vi "Flow Modelling_Comparison_Virtual Subjects_V2.4.1.vi"() -> ()   [LabVIEW 2017]
uses:
  <vilib>/Utility/file.llb/Read Delimited Spreadsheet (DBL).vi
  <vilib>/Analysis/NI_AALPro.lvlib
  <vilib>/gmath/NI_Gmath.lvlib
  <vilib>/Analysis/NI_AALBase.lvlib
  <vilib>/Analysis/baseanly.llb/Mean (DBL).vi
  <vilib>/Analysis/NI_AAL_SigProc.lvlib
panel:
  out "Array":dbl[][](array[numeric])
  out "mean 2":dbl
  out "SDW ZC 2":dbl
  out "mean":dbl
  in  "Min seperation B/W peaks":dbl format="%#_13g"
  out "intercept":dbl
  out "slope":dbl
  out "A1/A2":dbl
  out "Age (years)":dbl=75.0
  out "True - Type A or B":bool
  in  "Save Data":bool
  out "Saving Data":bool
  out "Loop time (ms)":u32=22
  in  "Loop Condition":bool
  in  "Loop Wait Time (ms)":u32
  in  "Start Subject ID":i32=1
  in  "Last Sub ID":i32=1000
  out "Current ID":i32=4341
  in  "Tab Control":T1(tab)
  out "Flow Rate":waveform(dbl)(graph)={"t0"=timestamp(0 s since 1904-01-01), "dt"=0.002, "Y"=array[402 elements]}
  in  "FileName P":string(combo)="PWs_Carotid_P.csv"
  in  "Param Folder Path":path=path "F:/HTIC Works/Cardiovascular Research/Data Set/Virtual Subjects Database"
  in  "Folder  Path":path=path "F:/HTIC Works/Cardiovascular Research/Data Set/Virtual Subjects Database/Virtual Subjects Database CSV"
  out "Hemodynamic Param":dbl[](array[numeric])=[75.0, 74.442, 66.405, 4.9433, 302.0, 1083.3, 80.0, 0.71264, 142.52, 52.007, 95.245, 90.517, 145.8, 50.057, 94.967, 95.743, 1.0577, 44.782, 49.473, 62.0, 12.106, 12.84, 15.216, 14.693, 38.642, 25.707, 15.209, 9.2134, 112.02, 2.665, 7.9438, 154.14]
  in  "Original Sampling Rate (Hz)":dbl=500.0
  in  "Re Sample?":bool
  out "dt":dbl=0.002
  in  "Re Sample Rate(Hz)":dbl=500.0 format="%#_13g"
  out "Pressure":waveform(dbl)(graph)={"t0"=timestamp(0 s since 1904-01-01), "dt"=0.002, "Y"=array[402 elements]}
  in  "FileName U":string(combo)="PWs_Carotid_U.csv"
  in  "FileName A":string(combo)="PWs_Carotid_A.csv"
  in  "FileName PPG":string(combo)="PWs_Carotid_PPG.csv"
  out "Flow Velocity":waveform(dbl)(graph)={"t0"=timestamp(0 s since 1904-01-01), "dt"=0.002, "Y"=array[402 elements]}
  out "Diameter":waveform(dbl)(graph)={"t0"=timestamp(0 s since 1904-01-01), "dt"=0.002, "Y"=array[402 elements]}
  out "PPG":waveform(dbl)(graph)={"t0"=timestamp(0 s since 1904-01-01), "dt"=0.002, "Y"=array[402 elements]}
  in  "FileName Param":string(combo)="pwdb_haemod_params.csv"
  out "Area":waveform(dbl)(graph)={"t0"=timestamp(0 s since 1904-01-01), "dt"=0.002, "Y"=array[402 elements]}
  in  "File to Save Data":path=path "F:/HTIC Works/Cardiovascular Research/Analysis and Results/Flow Model Comparison Virtual Subjects/Journal Data Analysis V2.0/Carotid_Flow_2_Ray_Type_Based_Master_0001_1000.xlsx" caption="Filename"
  out "Derivatives of P(t) 2":dynamicdata(graph)=[{"t0"=timestamp(0 s since 1904-01-01), "dt"=0.002, "Y"=array[402 elements]}, {"t0"=timestamp(0 s since 1904-01-01), "dt"=0.002, "Y"=array[402 elements]}, {"t0"=timestamp(0 s since 1904-01-01), "dt"=0.002, "Y"=array[402 elements]}, {"t0"=timestamp(0 s since 1904-01-01), "dt"=0.002, "Y"=array[402 elements]}, {"t0"=timestamp(0 s since 1904-01-01), "dt"=0.002, "Y"=array[402 elements]}, {"t0"=timestamp(0 s since 1904-01-01), "dt"=0.002, "Y"=[nan, nan, nan, nan, nan, 58.29028179551122, nan, nan, nan, nan, nan, nan, nan, nan, nan, nan, nan, 82.59575810473817, nan, nan, 88.92912718204488, 91.05758354114712, nan, nan, nan, nan, nan, nan, nan, nan, nan, nan, nan, nan, nan, nan, nan, nan, nan, nan, nan, 118.08771072319202, nan, nan, nan, 121.945536159601, nan, nan, nan, nan, nan, nan, nan, nan, nan, nan, nan, nan, nan, nan, nan, nan, nan, nan, nan, nan, nan, nan, nan, nan, nan, nan, nan, nan, nan, nan, nan, nan, nan, nan, nan, nan, nan, nan, nan, nan, nan, nan, nan, nan, nan, nan, nan, 143.88944139650874, 143.89889775561096, nan, nan, nan, nan, nan, nan, nan, nan, nan, nan, nan, nan, nan, nan, nan, nan, nan, nan, nan, nan, nan, nan, nan, nan, nan, nan, nan, nan, nan, nan, nan, nan, nan, nan, nan, nan, nan, nan, nan, nan, nan, nan, nan, nan, nan, nan, nan, nan, nan, nan, nan, nan, nan, nan, nan, nan, nan, nan, nan, nan, nan, nan, nan, nan, nan, 114.8030174563591, nan, nan, nan, nan, nan, nan, nan, nan, nan, nan, nan, nan, nan, nan, nan, nan, nan, nan, nan, nan, nan, nan, nan, nan, nan, nan, nan, nan, nan, nan, nan, nan, nan, nan, nan, nan, nan, nan, nan, nan, nan, nan, nan, nan, nan, nan, nan, nan, nan, nan, nan, nan, nan, nan, nan, nan, nan, nan, nan, nan, nan, nan, nan, nan, nan, nan, nan, nan, nan, nan, nan, nan, nan, nan, nan, nan, nan, nan, nan, nan, nan, nan, nan, nan, nan, nan, nan, nan, nan, nan, nan, nan, nan, nan, nan, nan, nan, nan, nan, nan, nan, nan, nan, nan, nan, nan, nan, nan, nan, nan, nan, nan, nan, nan, nan, nan, nan, nan, nan, nan, nan, nan, nan, nan, nan, nan, nan, nan, nan, nan, nan, nan, nan, nan, nan, nan, nan, nan, nan, nan, nan, nan, nan, nan, nan, nan, nan, nan, nan, nan, nan, nan, nan, nan, nan, nan, nan, nan, nan, nan, nan, nan, nan, nan, nan, nan, nan, nan, nan, nan, nan, nan, nan, nan, nan, nan, nan, nan, nan, nan, nan, nan, nan, nan, nan, nan, nan, nan, nan, nan, nan, nan, nan, nan, nan, nan, nan, nan, nan, nan, nan, nan, nan, nan, nan, nan, nan, nan, nan, nan, nan, nan, nan, nan, nan, nan, nan, nan, nan, nan, nan, nan, nan, nan, nan, nan, nan, nan, nan, nan, nan, nan, nan, nan, nan, nan, nan, nan, nan, nan, nan]}]
  in  "Derivative LPF cutoff (Hz)":dbl=75.0
  in  "SG Filter Config":T2={"polynomial order"=4, "side points"=28.0}
  out "Derivatives of P(t)":dynamicdata(graph)=[{"t0"=timestamp(0 s since 1904-01-01), "dt"=0.002, "Y"=array[402 elements]}, {"t0"=timestamp(0 s since 1904-01-01), "dt"=0.002, "Y"=array[401 elements]}, {"t0"=timestamp(0 s since 1904-01-01), "dt"=0.002, "Y"=array[401 elements]}, {"t0"=timestamp(0 s since 1904-01-01), "dt"=0.002, "Y"=array[401 elements]}, {"t0"=timestamp(0 s since 1904-01-01), "dt"=0.002, "Y"=array[402 elements]}, {"t0"=timestamp(0 s since 1904-01-01), "dt"=0.002, "Y"=[nan, nan, nan, nan, nan, 58.29028179551122, nan, nan, nan, nan, nan, nan, nan, nan, nan, nan, nan, 82.59575810473817, nan, nan, 88.92912718204488, 91.05758354114712, nan, nan, nan, nan, nan, nan, nan, nan, nan, nan, nan, nan, nan, nan, nan, nan, nan, nan, nan, 118.08771072319202, nan, nan, nan, 121.945536159601, nan, nan, nan, nan, nan, nan, nan, nan, nan, nan, nan, nan, nan, nan, nan, nan, nan, nan, nan, nan, nan, nan, nan, nan, nan, nan, nan, nan, nan, nan, nan, nan, nan, nan, nan, nan, nan, nan, nan, nan, nan, nan, nan, nan, nan, nan, nan, 143.88944139650874, 143.89889775561096, nan, nan, nan, nan, nan, nan, nan, nan, nan, nan, nan, nan, nan, nan, nan, nan, nan, nan, nan, nan, nan, nan, nan, nan, nan, nan, nan, nan, nan, nan, nan, nan, nan, nan, nan, nan, nan, nan, nan, nan, nan, nan, nan, nan, nan, nan, nan, nan, nan, nan, nan, nan, nan, nan, nan, nan, nan, nan, nan, nan, nan, nan, nan, nan, nan, 114.8030174563591, nan, nan, nan, nan, nan, nan, nan, nan, nan, nan, nan, nan, nan, nan, nan, nan, nan, nan, nan, nan, nan, nan, nan, nan, nan, nan, nan, nan, nan, nan, nan, nan, nan, nan, nan, nan, nan, nan, nan, nan, nan, nan, nan, nan, nan, nan, nan, nan, nan, nan, nan, nan, nan, nan, nan, nan, nan, nan, nan, nan, nan, nan, nan, nan, nan, nan, nan, nan, nan, nan, nan, nan, nan, nan, nan, nan, nan, nan, nan, nan, nan, nan, nan, nan, nan, nan, nan, nan, nan, nan, nan, nan, nan, nan, nan, nan, nan, nan, nan, nan, nan, nan, nan, nan, nan, nan, nan, nan, nan, nan, nan, nan, nan, nan, nan, nan, nan, nan, nan, nan, nan, nan, nan, nan, nan, nan, nan, nan, nan, nan, nan, nan, nan, nan, nan, nan, nan, nan, nan, nan, nan, nan, nan, nan, nan, nan, nan, nan, nan, nan, nan, nan, nan, nan, nan, nan, nan, nan, nan, nan, nan, nan, nan, nan, nan, nan, nan, nan, nan, nan, nan, nan, nan, nan, nan, nan, nan, nan, nan, nan, nan, nan, nan, nan, nan, nan, nan, nan, nan, nan, nan, nan, nan, nan, nan, nan, nan, nan, nan, nan, nan, nan, nan, nan, nan, nan, nan, nan, nan, nan, nan, nan, nan, nan, nan, nan, nan, nan, nan, nan, nan, nan, nan, nan, nan, nan, nan, nan, nan, nan, nan, nan, nan, nan, nan, nan, nan, nan, nan, nan, nan]}]
  out "Fid. Points":T3={"MX (sec)"=0.188, "FDW/SDW ZC (sec)"=0.058, "FoDW ZC (sec)"=0.12, "IP (sec)"=0.23573963204691295, "DN (sec)"=0.3188943360526481}
  out "True Flow Peak (sec)":dbl=0.042
  out "Peak of FoDW":dbl[](array[numeric])
  out "Fid. Points (SDW)":T4
  out "Zc (mmHg/ml/s)":dbl=1.725966148386607
  out "PVR (mmHg/ml/s)":dbl=16.50058753410355
  out "Input Impedence - Phase Spectrum":waveform(dbl)(graph)={"t0"=timestamp(0 s since 1904-01-01), "dt"=1.243781094527363, "Y"=array[402 elements]}
  out "Input Impedence - Magnitude Spectrum":waveform(dbl)(graph)={"t0"=timestamp(0 s since 1904-01-01), "dt"=1.243781094527363, "Y"=array[402 elements]}
  in  "Settings":T5={"Min. Harmonics for Zc"=4.0, "Max. Harmonics for Zc"=10.0}
  out "PWV (dPdU) (m/s)":dbl=21.61401999257581
  out "PWV (BH) (m/s)":dbl=13.16463528929057
  out "Zc (mmHg/ml/s)":dbl=2.673030331101323
  out "Zc (mmHg/ml/s)":dbl=1.6280853556278632
  in  "Settings 2":T6={"Min. Hrmonic for Zc"=4.0, "Max. Harmonic for Zc"=10.0}
  out "Input Impedence - Magnitude Spectrum  2":waveform(dbl)(graph)={"t0"=timestamp(0 s since 1904-01-01), "dt"=1.243781094527363, "Y"=array[402 elements]}
  out "WSA Q - Time Domain":dynamicdata(graph)=[{"t0"=timestamp(0 s since 1904-01-01), "dt"=0.002, "Y"=array[402 elements]}, {"t0"=timestamp(0 s since 1904-01-01), "dt"=0.002, "Y"=array[402 elements]}, {"t0"=timestamp(0 s since 1904-01-01), "dt"=0.002, "Y"=array[402 elements]}]
  out "WSA P - Time. Domain":dynamicdata(graph)=[{"t0"=timestamp(0 s since 1904-01-01), "dt"=0.002, "Y"=array[402 elements]}, {"t0"=timestamp(0 s since 1904-01-01), "dt"=0.002, "Y"=array[402 elements]}, {"t0"=timestamp(0 s since 1904-01-01), "dt"=0.002, "Y"=array[402 elements]}]
  out "WSA Q - Freq. Domain":dynamicdata(graph)=[{"t0"=timestamp(0 s since 1904-01-01), "dt"=0.002, "Y"=array[402 elements]}, {"t0"=timestamp(0 s since 1904-01-01), "dt"=0.002, "Y"=array[402 elements]}, {"t0"=timestamp(0 s since 1904-01-01), "dt"=0.002, "Y"=array[402 elements]}]
  out "WSA P - Freq. Domain":dynamicdata(graph)=[{"t0"=timestamp(0 s since 1904-01-01), "dt"=0.002, "Y"=array[402 elements]}, {"t0"=timestamp(0 s since 1904-01-01), "dt"=0.002, "Y"=array[402 elements]}, {"t0"=timestamp(0 s since 1904-01-01), "dt"=0.002, "Y"=array[402 elements]}]
  out "Reflection Markers\n(Time Domain WSA)":T7={"del Pf"=58.89527020287039, "del Pb"=41.94891474189147, "RM"=0.7122628794705317, "RI (%)"=41.59775277560059}
  out "Reflection Markers\n(Freq. Domain WSA)":T7={"del Pf"=54.396213288918176, "del Pb"=39.3327759196838, "RM"=0.7230793016928043, "RI (%)"=41.96436582938637}
  out "m-Ray":dbl[][](graph)
  out "Magnitude Spectrum Flow":dynamicdata(graph)=[{"t0"=timestamp(0 s since 1904-01-01), "dt"=1.243781094527363, "Y"=array[201 elements]}, {"t0"=timestamp(0 s since 1904-01-01), "dt"=1.2468827930174562, "Y"=[2.875475307707561, 3.6127603544098683, 2.601261591287198, 1.6917776838030885, 1.1941771538443262, 0.9487554465134683, 0.7694402798879594, 0.6103288199328872, 0.4731880654990021, 0.36211255149969857, 0.2769548748250606, 0.21434413683079837, 0.1694301710225544, 0.13733282803274616, 0.11402801928183168, 0.09662400462795698, 0.08321657451570393, 0.07259766150124436, 0.0639964187444626, 0.056904741290042034, 0.050973683000770764, 0.04595437718864926, 0.041663805403745764, 0.037964077971374716, 0.03474926453416704, 0.031936660619215164, 0.029460797434445064, 0.027269222135548016, 0.025319459881613045, 0.023576786205464897, 0.022012567439413037, 0.020603006949110554, 0.019328186072354925, 0.018171322213655604, 0.017118189050174, 0.016156659190830255, 0.015276340329362368, 0.014468283485487652, 0.013724747334456168, 0.013039006543154078, 0.012405194902865806, 0.011818176176362818, 0.011273437168463712, 0.010766998730631047, 0.010295341324676783, 0.009855342472415885, 0.009444223960556648, 0.009059507092347416, 0.008698974608396304, 0.008360638159887837, 0.008042710424359204, 0.007743581119138634, 0.0074617962998756145, 0.007196040438151105, 0.006945120858491341, 0.006707954185289361, 0.006483554507505954, 0.00627102301606209, 0.006069538907604141, 0.005878351380350117, 0.005696772574338759, 0.005524171330542793, 0.005359967661818076, 0.0052036278441806956, 0.00505466004996289, 0.0049126104554011564, 0.0047770597645341445, 0.004647620099193955, 0.004523932211592496, 0.004405662981762424, 0.004292503166987805, 0.004184165374607464, 0.004080382233152479, 0.00398090473991798, 0.0038855007657562566, 0.0037939537001872204, 0.003706061221966357, 0.0036216341819848476, 0.003540495586902267, 0.0034624796732586217, 0.003387431062954797, 0.0033152039920320057, 0.003245661605543917, 0.003178675312137021, 0.0031141241926116317, 0.0030518944573612915, 0.002991878948129061, 0.0029339766799803533, 0.002878092419823849, 0.0028241362981836623, 0.0027720234512541744, 0.002721673690565746, 0.002673011197849946, 0.002625964242935183, 0.0025804649226975913, 0.0025364489192982675, 0.0024938552760841457, 0.002452626189704618, 0.0024127068171034462, 0.002374045096189568, 0.0023365915790872476, 0.00230029927696597, 0.0022651235155401643, 0.00223102180040995, 0.002197953691483903, 0.0021658806857857635, 0.0021347661080214518, 0.0021045750083141137, 0.002075274066582661, 0.002046831503073918, 0.002019216994597034, 0.001992401596055293, 0.0019663576668881018, 0.0019410588020834878, 0.0019164797674358094, 0.0018925964387492304, 0.0018693857447258516, 0.0018468256132752187, 0.001824894921018906, 0.0018035734457731835, 0.0017828418218158767, 0.001762681497743173, 0.0017430746967612542, 0.0017240043792384348, 0.0017054542073845459, 0.0016874085119173083, 0.0016698522605864423, 0.001652771028445564, 0.0016361509697526123, 0.0016199787914136649, 0.0016042417278542903, 0.001588927517255393, 0.0015740243790484032, 0.0015595209926116604, 0.0015454064770874616, 0.00153167037225232, 0.001518302620390819, 0.0015052935490970777, 0.0014926338549648165, 0.0014803145881091097, 0.0014683271374716065, 0.0014566632168709034, 0.0014453148517466628, 0.0014342743665710113, 0.001423534372880088, 0.0014130877578963801, 0.0014029276737148768, 0.0013930475270104972, 0.0013834409692506475, 0.0013741018873806075, 0.0013650243949579809, 0.0013562028237132488, 0.001347631715514795, 0.001339305814715998, 0.001331220060867736, 0.0013233695817755878, 0.0013157496868858958, 0.0013083558609843034, 0.0013011837581918626, 0.0012942291962411733, 0.001287488151027233, 0.0012809567514092683, 0.0012746312742586898, 0.001268508139743941, 0.0012625839068313555, 0.0012568552690039238, 0.0012513190501797634, 0.0012459722008272467, 0.0012408117942623747, 0.0012358350231262449, 0.0012310391960329112, 0.0012264217343779297, 0.0012219801693055961, 0.0012177121388237048, 0.0012136153850642354, 0.0012096877516847855, 0.0012059271813955653, 0.0012023317136246772, 0.0011988994822993734, 0.001195628713749398, 0.0011925177247257275, 0.0011895649205306458, 0.0011867687932546778, 0.0011841279201161216, 0.0011816409619078844, 0.0011793066615325718, 0.0011771238426436684, 0.0011750914083724123, 0.0011732083401441626, 0.0011714736965906787, 0.0011698866125403051, 0.0011684462980971273, 0.0011671520378015504, 0.001166003189871259, 0.0011649991855236896, 0.0011641395283739614, 0.0011634237939147955, 0.001162851629066894, 0.0011624227518108622, 0.0011621369508905742]}, {"t0"=timestamp(0 s since 1904-01-01), "dt"=1.2468827930174562, "Y"=[3.7508500728179532, 4.5245622515687804, 2.7381315525642167, 1.2960200155292345, 1.0722958286591062, 0.8591503498715637, 0.5835761351400733, 0.5409096008292368, 0.4147688861808805, 0.32048488221512145, 0.29183680892133157, 0.20830482531413225, 0.17423818235279553, 0.14408511660630235, 0.09295183114010737, 0.08066585123213792, 0.05245806743771004, 0.02590171014916199, 0.020442136353742146, 0.009784595168948028, 0.011474868149847212, 0.018825340120545746, 0.03141941850998123, 0.02947371209902249, 0.03581015185540728, 0.03916182600261739, 0.034561584685847385, 0.03873980795285254, 0.03511313154107394, 0.03116123233701509, 0.031912924558875844, 0.02491230464070535, 0.022634935322990154, 0.020002838241100496, 0.012977935928489096, 0.011842854009855807, 0.007328558363566402, 0.002244810549003913, 0.0017397365874485381, 0.004532861640760953, 0.005726147321061923, 0.007405227865666979, 0.010966826405368063, 0.010414787796708059, 0.012306490583137283, 0.013401593295404544, 0.011949767607856616, 0.013387475714232414, 0.012171390141769123, 0.01081417184514539, 0.011125760149963679, 0.008526081768583077, 0.007706560831230049, 0.006699089826276321, 0.0039008866101970107, 0.003497414628569744, 0.001773368465099045, 0.00047989313530877586, 0.000946729075561772, 0.003251762903982372, 0.0038078559422530457, 0.004464019719007958, 0.006079369674982631, 0.005710634319960984, 0.006535479575465597, 0.006978137171141666, 0.006151608672064754, 0.006802070499646614, 0.006078711193183457, 0.00530783478093735, 0.005407263205985483, 0.003953597615943812, 0.0034948522720437136, 0.002903582890828807, 0.0013417822627342514, 0.0011393625525869247, 0.0005372069831318354, 0.0010815373739305463, 0.0012525598901868763, 0.002571610507446599, 0.002850884833977321, 0.003162498326287775, 0.004062517723188385, 0.0037524296049899404, 0.0041825485685056596, 0.004367767696673512, 0.0037782933874932045, 0.0041208391029226256, 0.0035852324475160046, 0.003052998354699827, 0.003063478402111416, 0.0020799201132795865, 0.0017818005793410658, 0.001359917731252523, 0.00033081700568838695, 0.0002472925184793049, 0.0006353239473414299, 0.001224390605035756, 0.001291746507604338, 0.002145466179865607, 0.002283235237248078, 0.0024430485314186428, 0.003006307934302749, 0.0027230010421153443, 0.0029731708270343696, 0.0030340432764327826, 0.002564428140558709, 0.002763719020567095, 0.0023209272461199855, 0.001917753419707948, 0.0018866915958778356, 0.001142184536290282, 0.0009435979213443637, 0.0006009834971304799, 0.00015563871856385234, 0.00025488504953471, 0.0007999141673041498, 0.0012400965762612182, 0.0012548964511063009, 0.0018618021285207076, 0.00191633817055137, 0.0019995049706351274, 0.002379614848642651, 0.0021097458485435615, 0.0022683889315689384, 0.0022593891694644755, 0.0018602703564758424, 0.001985640883157327, 0.0015932606855256976, 0.0012728288480013971, 0.0012185033302108954, 0.000609944887714449, 0.0004946215828014669, 0.00017913489638318402, 0.00041534120526386884, 0.00046290996057953346, 0.0008937400922277749, 0.0012240257805451386, 0.0012081530224320456, 0.0016724486765397817, 0.0016718389500814865, 0.0017138288795263978, 0.001984171073359226, 0.0017196672622895987, 0.001829264129194719, 0.001774799824540436, 0.0014202635123030359, 0.0015044633021834733, 0.0011381144596961585, 0.000877372347329584, 0.0008050885390449594, 0.000278499702809272, 0.0002698473312872596, 9.641728518399287e-05, 0.0005793341438433319, 0.0005960928699227096, 0.0009585113628025477, 0.0012121650203852962, 0.001177123910926902, 0.0015550836888611236, 0.0015134003492032705, 0.0015330199512812203, 0.001732245289408295, 0.0014663755863387655, 0.0015491377483849418, 0.0014597230614821599, 0.001133181926904543, 0.0011921630821759533, 0.0008345755925252025, 0.0006210987382223606, 0.0005288786284448412, 6.866564153260373e-05, 0.0002348812509856483, 0.0002819154758607105, 0.0007052224535725401, 0.0006992791072680399, 0.0010249158270583772, 0.0012232930978217363, 0.0011755815989433625, 0.0015004968361050067, 0.001423993327248736, 0.001431481248622589, 0.0015808000227044321, 0.0013062342066300684, 0.0013737589587263772, 0.0012521900650118711, 0.0009403417096469833, 0.0009811026261219574, 0.0006175136507945863, 0.00044542496927388764, 0.00032548202569685256, 0.00015424392272724206, 0.00031738262133868103, 0.00044468091725355797, 0.0008292865567833156, 0.0008050655206424677, 0.0011156902134628515, 0.0012719611413126496, 0.0012146041020032518, 0.0015074412858806026]}]
  out "RMSE Ray Model":dbl=4.137711413874004
  out "Model Error (ms)":dbl[](array[numeric])=[5.999999999999998, 4.029709151279315]
  out "Reference Flow Rate":T8={"Flow Peak (sec)"=0.042, "Flow Peak (Amp)"=18.5690232}
  out "Flow Rate Model":dynamicdata(graph)=[{"t0"=timestamp(0 s since 1904-01-01), "dt"=0.002, "Y"=array[402 elements]}, {"t0"=timestamp(0 s since 1904-01-01), "dt"=0.002, "Y"=[nan, nan, nan, nan, nan, nan, nan, nan, nan, nan, nan, nan, nan, nan, nan, nan, nan, nan, nan, nan, 88.92912718204488, nan, nan, nan, nan, nan, nan, nan, nan, nan, nan, nan, nan, nan, nan, nan, nan, nan, nan, nan, nan, nan, nan, nan, nan, nan, nan, nan, nan, nan, nan, nan, nan, nan, nan, nan, nan, nan, nan, nan, nan, nan, nan, nan, nan, nan, nan, nan, nan, nan, nan, nan, nan, nan, nan, nan, nan, nan, nan, nan, nan, nan, nan, nan, nan, nan, nan, nan, nan, nan, nan, nan, nan, nan, nan, nan, nan, nan, nan, nan, nan, nan, nan, nan, nan, nan, nan, nan, nan, nan, nan, nan, nan, nan, nan, nan, nan, nan, nan, nan, nan, nan, nan, nan, nan, nan, nan, nan, nan, nan, nan, nan, nan, nan, nan, nan, nan, nan, nan, nan, nan, nan, nan, nan, nan, nan, nan, nan, nan, nan, nan, nan, nan, nan, nan, nan, nan, nan, nan, nan, 114.8030174563591, nan, nan, nan, nan, nan, nan, nan, nan, nan, nan, nan, nan, nan, nan, nan, nan, nan, nan, nan, nan, nan, nan, nan, nan, nan, nan, nan, nan, nan, nan, nan, nan, nan, nan, nan, nan, nan, nan, nan, nan, nan, nan, nan, nan, nan, nan, nan, nan, nan, nan, nan, nan, nan, nan, nan, nan, nan, nan, nan, nan, nan, nan, nan, nan, nan, nan, nan, nan, nan, nan, nan, nan, nan, nan, nan, nan, nan, nan, nan, nan, nan, nan, nan, nan, nan, nan, nan, nan, nan, nan, nan, nan, nan, nan, nan, nan, nan, nan, nan, nan, nan, nan, nan, nan, nan, nan, nan, nan, nan, nan, nan, nan, nan, nan, nan, nan, nan, nan, nan, nan, nan, nan, nan, nan, nan, nan, nan, nan, nan, nan, nan, nan, nan, nan, nan, nan, nan, nan, nan, nan, nan, nan, nan, nan, nan, nan, nan, nan, nan, nan, nan, nan, nan, nan, nan, nan, nan, nan, nan, nan, nan, nan, nan, nan, nan, nan, nan, nan, nan, nan, nan, nan, nan, nan, nan, nan, nan, nan, nan, nan, nan, nan, nan, nan, nan, nan, nan, nan, nan, nan, nan, nan, nan, nan, nan, nan, nan, nan, nan, nan, nan, nan, nan, nan, nan, nan, nan, nan, nan, nan, nan, nan, nan, nan, nan, nan, nan, nan, nan, nan, nan, nan, nan, nan, nan, nan, nan, nan, nan, nan, nan, nan, nan, nan, nan, nan, nan, nan, nan, nan, nan]}, {"t0"=timestamp(0 s since 1904-01-01), "dt"=0.002, "Y"=array[402 elements]}, {"t0"=timestamp(0 s since 1904-01-01), "dt"=0.002, "Y"=array[401 elements]}, {"t0"=timestamp(0 s since 1904-01-01), "dt"=0.002, "Y"=array[401 elements]}, {"t0"=timestamp(0 s since 1904-01-01), "dt"=0.002, "Y"=array[401 elements]}]
  out "T_Ejection Period (sec)":dbl=0.31908927539190324
  out "T_Flow Peak (sec)":dbl=0.04
  out "Model Optimised Parameter":dbl[](array[numeric])=[0.10000000149011612, 0.03999999910593033]
  out "#Rayeligh":dbl=2.0
  out "correlation coefficient r":dbl=0.9951884045954855 format="%.7g"
  out "Amplitude":dbl[](array[numeric])
  out "A2/A1":dbl
  in  "A2/A1 2":dbl
  out "m-Ray RWTT XCorr (TD)(ms)":dbl=72.00000000000001
  out "Ref. RWTT XCorr (TD)(ms)":dbl=48.0
  out "Tri.  RWTT XCorr (TD)(ms)":dbl=84.0
  out "m-Ray RWTT XCorr (FD)(ms)":dbl=42.0
  out "Ref. RWTT XCorr (FD)(ms)":dbl=34.0
  out "Tri.  RWTT XCorr (FD)(ms)":dbl=48.0
  out "m-Ray RWTT ZC (TD)(ms)":dbl=72.41752223636087
  out "Ref. RWTT ZC (TD)(ms)":dbl=48.9881513554138
  out "Tri.  RWTT  ZC (TD)(ms)":dbl=79.1625821471164
  out "m-Ray RWTT ZC (FD)(ms)":dbl=46.35509024365538
  out "Ref. RWTT ZC (FD)(ms)":dbl=36.51530586869714
  out "Tri.  RWTT ZC (FD)(ms)":dbl=48.6059655733487
  out "RMSE (Fwd Triangular TD)":dbl=3.386520035598584
  out "RMSE (Bwd Rayleigh TD)":dbl=3.726988173192518
  out "RMSE (Fwd Rayleigh TD)":dbl=3.726988173192517
  out "RMSE (Bwd Triangular TD)":dbl=3.3865200355985845
  out "Backward Pressure Wave (Time Domain Analysis)":dynamicdata(graph)=[{"t0"=timestamp(0 s since 1904-01-01), "dt"=0.002, "Y"=array[402 elements]}, {"t0"=timestamp(0 s since 1904-01-01), "dt"=0.002, "Y"=array[401 elements]}, {"t0"=timestamp(0 s since 1904-01-01), "dt"=0.002, "Y"=array[401 elements]}]
  out "Forward Pressure Wave (Time Domain Analysis)":dynamicdata(graph)=[{"t0"=timestamp(0 s since 1904-01-01), "dt"=0.002, "Y"=array[402 elements]}, {"t0"=timestamp(0 s since 1904-01-01), "dt"=0.002, "Y"=array[401 elements]}, {"t0"=timestamp(0 s since 1904-01-01), "dt"=0.002, "Y"=array[401 elements]}]
  out "Rayleigh (FD)":T7={"del Pf"=50.48708754008288, "del Pb"=45.11476622884561, "RM"=0.8935901916114282, "RI (%)"=47.19026300252385}
  out "Triangular (FD)":T7={"del Pf"=54.83519661326886, "del Pb"=40.555492402948346, "RM"=0.739588711406842, "RI (%)"=42.51514777931164}
  out "Reference (FD)":T7={"del Pf"=54.396213288918176, "del Pb"=39.3327759196838, "RM"=0.7230793016928043, "RI (%)"=41.96436582938637}
  out "RMSE (Fwd Triangular FD)":dbl=1.7174517386171273
  out "RMSE (Bwd Rayleigh FD)":dbl=2.4763715027755246
  out "RMSE (Fwd Rayleigh FD)":dbl=2.476371502775524
  out "RMSE (Bwd Triangular FD)":dbl=1.7174517386171277
  out "Backward Pressure Wave (Freq. Domain Analysis)":dynamicdata(graph)=[{"t0"=timestamp(0 s since 1904-01-01), "dt"=0.002, "Y"=array[402 elements]}, {"t0"=timestamp(0 s since 1904-01-01), "dt"=0.002, "Y"=array[401 elements]}, {"t0"=timestamp(0 s since 1904-01-01), "dt"=0.002, "Y"=array[401 elements]}]
  out "Forward Pressure Wave (Freq. Domain Analysis)":dynamicdata(graph)=[{"t0"=timestamp(0 s since 1904-01-01), "dt"=0.002, "Y"=array[402 elements]}, {"t0"=timestamp(0 s since 1904-01-01), "dt"=0.002, "Y"=array[401 elements]}, {"t0"=timestamp(0 s since 1904-01-01), "dt"=0.002, "Y"=array[401 elements]}]
  out "CO (l/min)":dbl=4.9433
  out "SV (ml)":dbl=66.405
  out "cf-PWV (m/s)":dbl=12.84
  out "Aortic PWV (m/s)":dbl=12.106
  out "Tr (ms)":dbl=62.0
  out "AIx (%)":dbl=49.473
  out "AP (mmHg)":dbl=44.782
  out "PWV (BH)":dbl=9.950315267478873
  out "AC":dbl=0.3558142554910398
  out "Ep":dbl=367.41215927607345
  out "Beta":dbl=30.70141582661549
  out "AIx":T9={"Type (4th D ZC)"=enum."Type A", "AIx (%) (4th D ZC) "=27.868164767546343, "AP (mmHg)  (4th DZC)"=25.811187032418943}
  out "SBP (mmHg)":dbl=143.89889775561096
  out "DBP (mmHg)":dbl=51.28
  out "Triangular (TD)":T7={"del Pf"=63.05128557028921, "del Pb"=45.2280154011999, "RM"=0.7173210663687415, "RI (%)"=41.769770395090404}
  out "Rayleigh (TD)":T7={"del Pf"=55.90262934015283, "del Pb"=50.81292933822665, "RM"=0.9089541929958842, "RI (%)"=47.61529618316221}
  out "Reference (TD)":T7={"del Pf"=58.89527020287039, "del Pb"=41.94891474189147, "RM"=0.7122628794705317, "RI (%)"=41.59775277560059}
  out "PVR (mmHg/ml/s) - Reference":dbl=16.50058753410355
  out "PVR (mmHg/ml/s) - Rayleigh":dbl=33.19021836521006
  out "PVR (mmHg/ml/s) - Triangular":dbl=25.44427303512101
  out "Zc TD (mmHg/ml/s) - Triangular":dbl=3.0721951458665524
  out "Zc TD (mmHg/ml/s) - Reference":dbl=2.673030331101323
  out "Zc TD (mmHg/ml/s) - Rayleigh":dbl=2.834159231448205
  out "Zc FD (mmHg/ml/s) - Reference":dbl=1.725966148386607
  out "Zc FD (mmHg/ml/s) - Rayleigh":dbl=1.48764333842042
  out "Zc FD (mmHg/ml/s) - Triangular":dbl=1.702280253067496
  out "A2/A1 vs. AIx":cluster{dbl[], "Best Linear Fit":dbl[]}[](graph)
  out "A2/A1 vs Age":cluster{dbl[], "Best Linear Fit":dbl[]}[](graph)
  out "XY Graph 3":cluster{dbl[], dbl[]}(graph)
  out "correlation coefficient r 3":dbl format="%.7g"
  out "XY Graph 2":cluster{dbl[], dbl[]}(graph)
  out "XY Graph":cluster{dbl[], dbl[]}(graph)
  out "correlation coefficient r 2":dbl format="%.7g"
  out "mean RMSE for Q":dbl format="%0.2f"
  out "mean Peak err":dbl format="%0.2f"
  out "mean base err":dbl format="%0.2f"
  out "mean RMSE PF":dbl format="%0.2f"
  out "mean RMSE PB":dbl format="%0.2f"
  # "VIRTUAL SUBJECTS DATABASE PLATFORM FOR PULSE WAVE ANALYSIS"
  # "SETTINGS"
  # "PULSE CONTOUR MARKERS"
  # "CHARACTERISTIC IMPEDENCE\n FREQUENCY DOMAIN ANALYSIS"
  # "CHARACTERISTIC IMPEDENCE\n TIME DOMAIN ANALYSIS"
  # "CLASSICAL WAVE SEPERATION ANALYSIS"
  # "REFLECTION MARKERS"
  # "Peak Error"
  # "Base Error"
  # "Parameters\nfrom Database"
  # "STIFFNESS MARKERS"
  # "IMPEDANCE ANALYSIS- PVR and ZC"
  # "ERROR ANALYSIS"
  # "REFLECTION QUANTIFICATION"
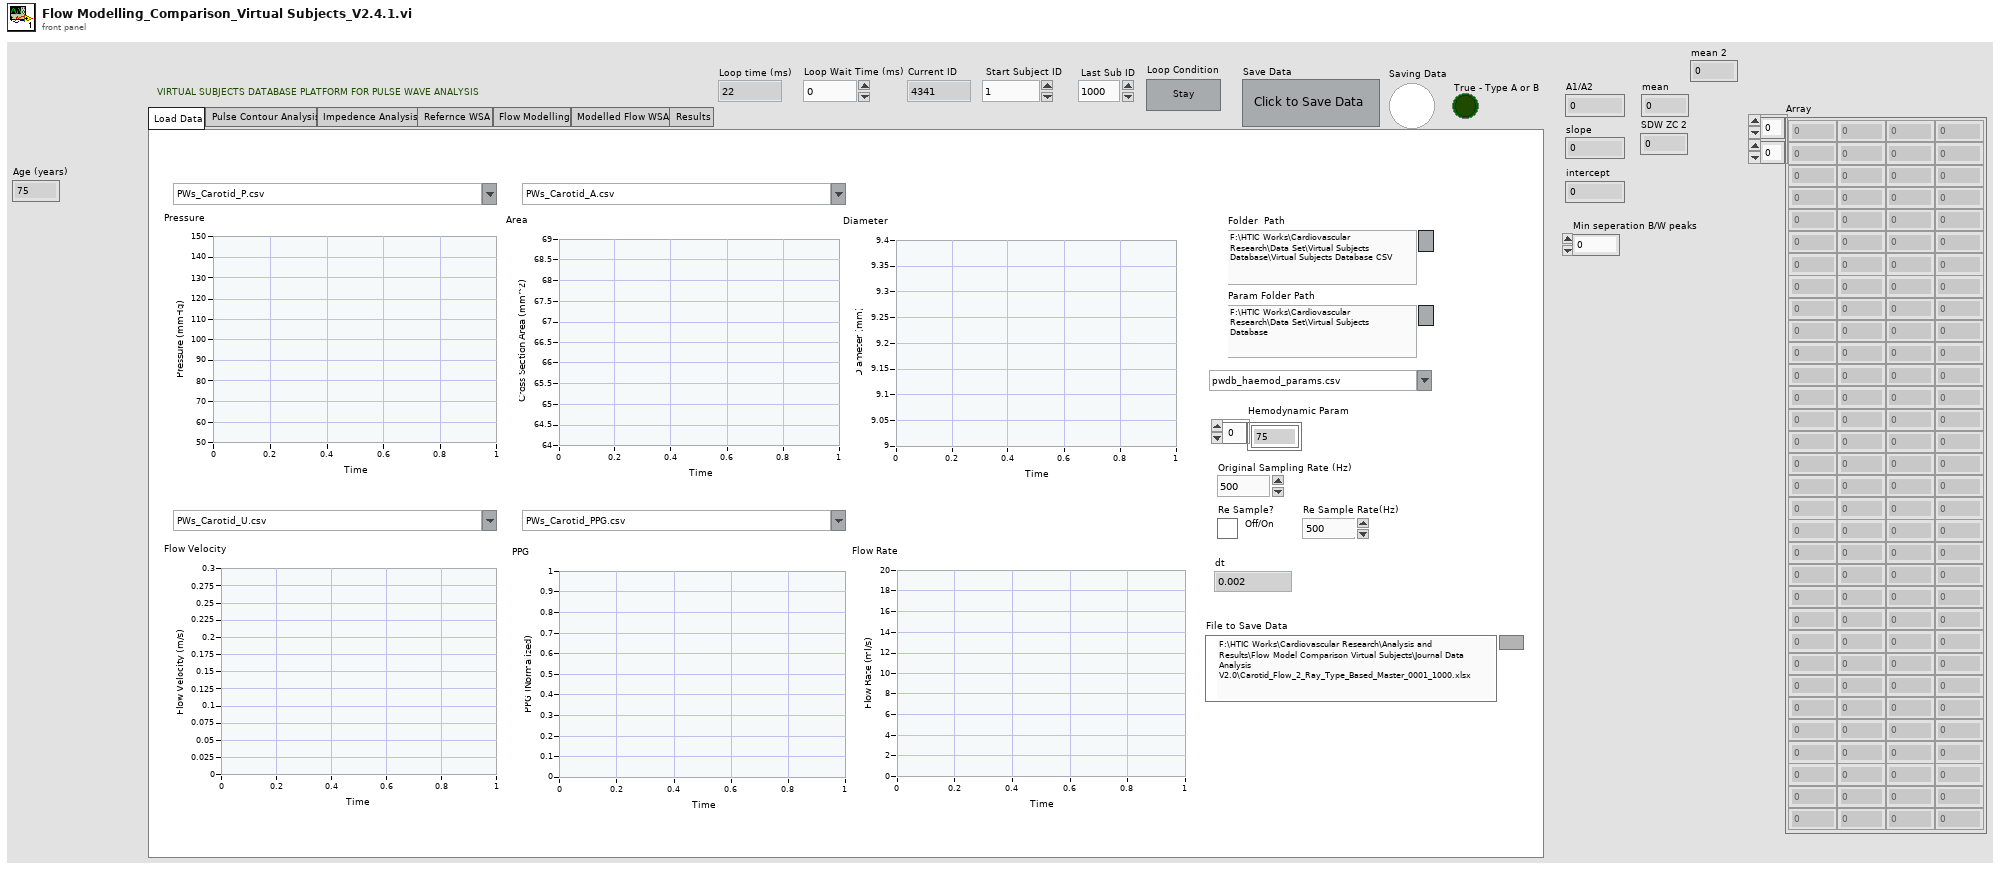
[diagram p1: front panel]
types:
  T1 = enum32{"Load Data", "Pulse Contour Analysis", "Impedence Analysis", "Refernce WSA", "Flow Modelling", "Modelled Flow WSA", "Results"}
  T2 = cluster{"polynomial order":i32, "side points":dbl}
  T3 = cluster{"MX (sec)":dbl, "FDW/SDW ZC (sec)":dbl, "FoDW ZC (sec)":dbl, "IP (sec)":dbl, "DN (sec)":dbl}
  T4 = cluster{"SF":dbl, "ER":dbl, "IP":dbl, "DN":dbl, "SDW ZC 1":dbl, "MX":dbl, "FDW ZC":dbl, "FoDW ZC":dbl, "SDW ZC 2":dbl}
  T5 = cluster{"Min. Harmonics for Zc":dbl, "Max. Harmonics for Zc":dbl}
  T6 = cluster{"Min. Hrmonic for Zc":dbl, "Max. Harmonic for Zc":dbl}
  T7 = cluster{"del Pf":dbl, "del Pb":dbl, "RM":dbl, "RI (%)":dbl}
  T8 = cluster{"Flow Peak (sec)":dbl, "Flow Peak (Amp)":dbl}
  T9 = cluster{"Type (4th D ZC)":enum16{"Type A", "Type B", "Type C"}, "AIx (%) (4th D ZC) ":dbl, "AP (mmHg)  (4th DZC)":dbl}
  T10 = cluster{"Pressure (mmHg)":waveform(dbl), "Area (mm^2)":waveform(dbl), "Flow Velocity (m/s)":waveform(dbl), "Flow Rate (ml/s)":waveform(dbl), "Diameter (mm)":waveform(dbl), "PPG":waveform(dbl)}
  T11 = enum16{"STOP", "5-Rayleigh Model", "4-Rayeligh Model", "3-Rayleigh Model", "2-Rayleigh Model", "1-Rayleigh Model"}
  T12 = cluster{"MX (s)":dbl, "SD ZC 1 (s)":dbl, "FoDW ZC (s)":dbl, "IP (s)":dbl, "DN (s)":dbl, "SD ZC 2( s)":dbl}
  T13 = cluster{"FDW":waveform(dbl), "SDW":waveform(dbl), "FoDW":waveform(dbl)}
  T14 = cluster{"P FWD":waveform(dbl), "P BWD":waveform(dbl), "Q FWD":waveform(dbl), "Q BWD":waveform(dbl)}
  T15 = cluster{"del Pf (mmHg)":dbl, "del Pb (mmHg)":dbl, "RM":dbl, "RI (%)":dbl}
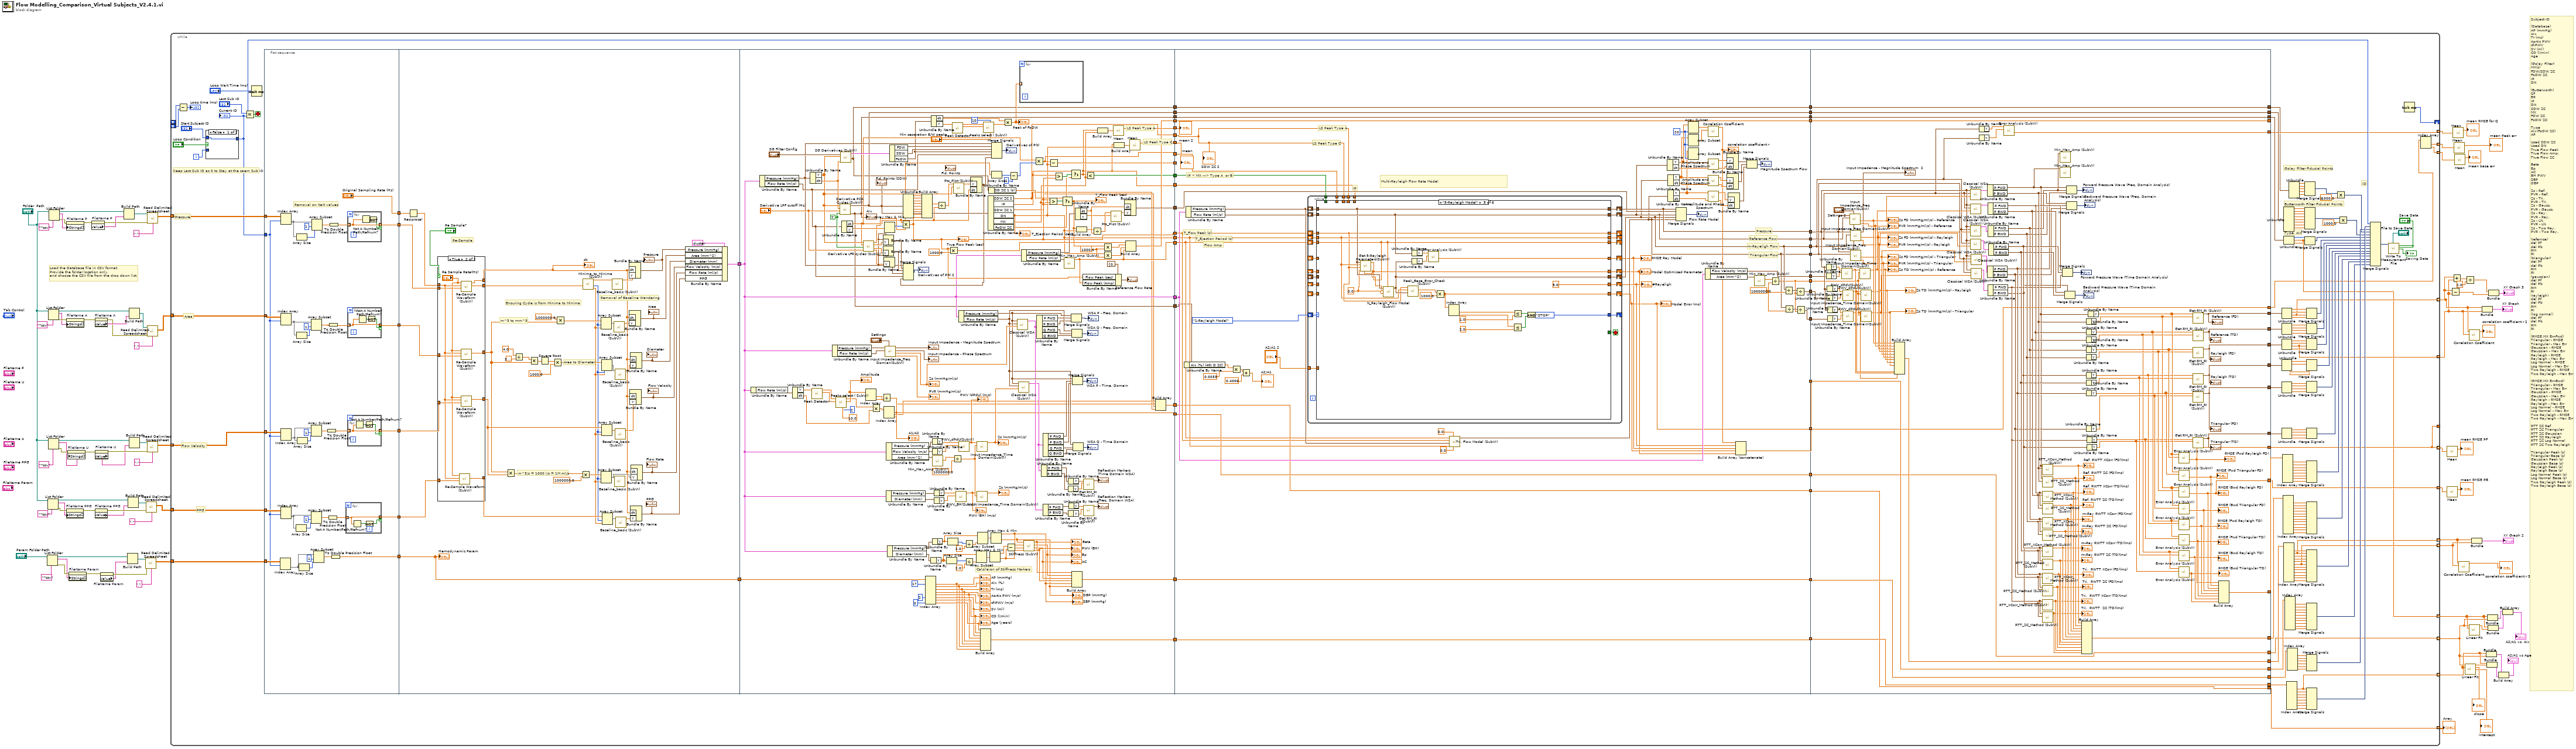
[diagram p0: block diagram]
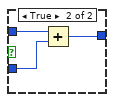
[diagram p2: hidden frame]
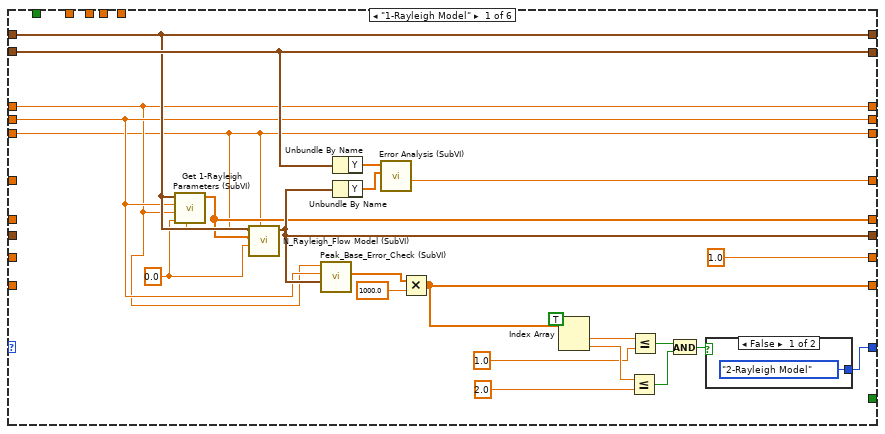
[diagram p4: hidden frame]
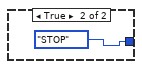
[diagram p5: hidden frame]
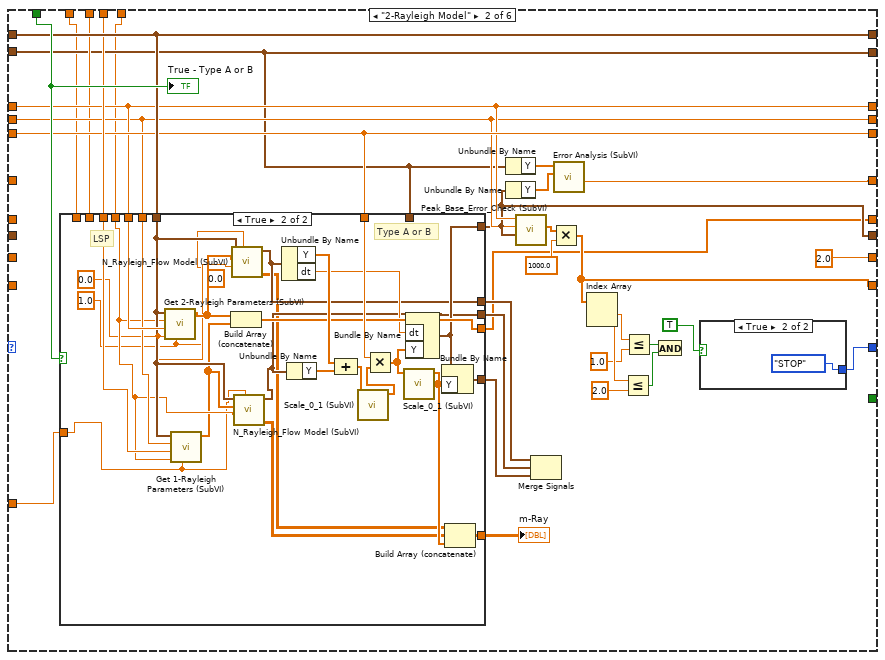
[diagram p6: hidden frame]
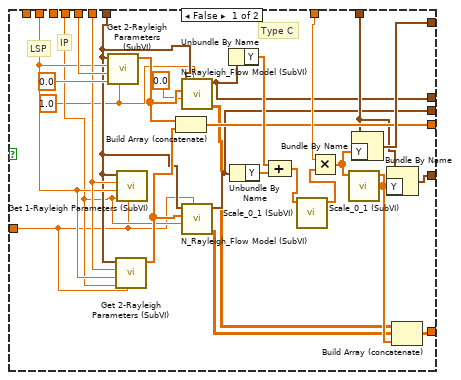
[diagram p7: hidden frame]
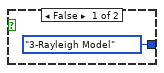
[diagram p8: hidden frame]
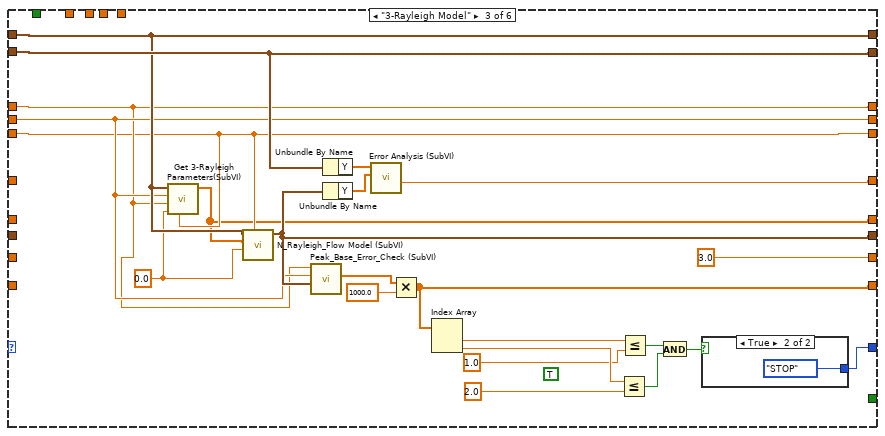
[diagram p9: hidden frame]
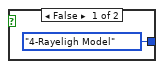
[diagram p10: hidden frame]
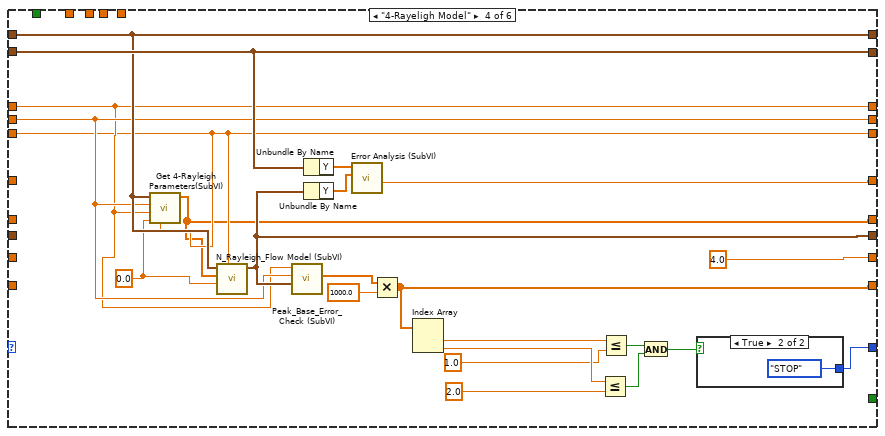
[diagram p11: hidden frame]
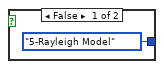
[diagram p12: hidden frame]
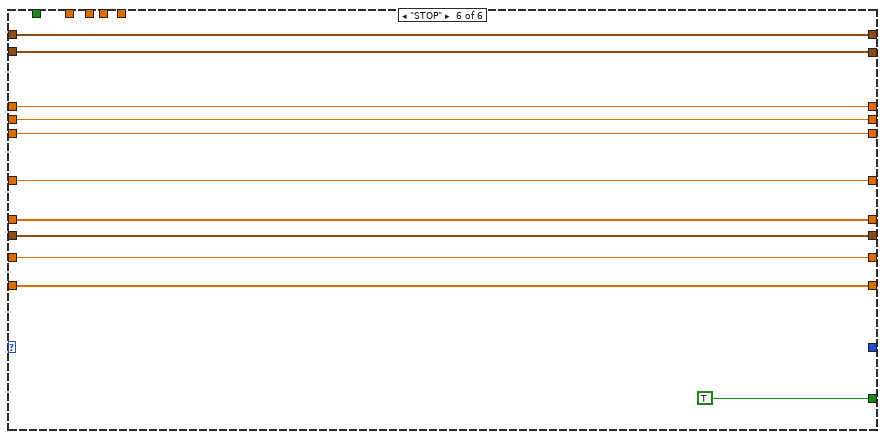
[diagram p13: hidden frame]
diagram:
  # "Subject ID\n\n(Database)\nAP (mmHg)\nAIx\nTr (ms)\nAortic PWV\ncf-PWV\nSV (ml)\nCO (l/min)\nAge\n\n(Golay Filter)\nMX(s)\nFDW/SDW ZC\nFoDW ZC\nIP\nDN\n\n(Butterworth)\nSF\nER\nIP\nDN\nSDW ZC\nMX\nFDW ZC\nFoDW ZC\n\nType\nAIx(FoDW ZC)\nAP\n\nUsed SDW ZC\nUsed DN\nTrue Flow Peak\nTrue Flow Amp.\nTrue Flow ZC\n\nBeta\nEp\nAC\nBH PWV\nSBP\nDBP\n\nZc - Ref.\nPVR - Ref.\nZc - Tri.\nPVR - Tri.\nZc - Gauss.\nPVR - Gauss.\nZc - Ray.\nPVR - Ray.\nZc - LN.\nPVR - LN.\nZc - Two Ray.\nPVR - Two Ray.\n\n(refernce)\ndel Pf\ndel Pb\nRM\nRI\n(triangular)\ndel Pf\ndel Pb\nRM\nRI\n(gaussian)\ndel Pf\ndel Pb\nRM\nRI\n(rayleigh)\ndel Pf\ndel Pb\nRM\nRI\n(log normal)\ndel Pf\ndel Pb\nRM\nRI\n\n(RMSE,MX Err-Fwd)\nTriangular - RMSE\nTriangular - Max Err\nGaussian - RMSE\nGaussian - Max Err\nRayleigh - RMSE\nRayleigh - Max Err\nLog Normal - RMSE\nLog Normal - Max Err\nTwo Rayleigh - RMSE\nTwo Rayleigh - Max Err\n\n(RMSE,MX Err-Bwd)\nTriangular - RMSE\nTriangular - Max Err\nGaussian - RMSE\nGaussian - Max Err\nRayleigh - RMSE\nRayleigh - Max Err\nLog Normal - RMSE\nLog Normal - Max Err\nTwo Rayleigh - RMSE\nTwo Rayleigh - Max Err\n\nRTT ZC Ref\nRTT ZC Triangular\nRTT ZC Gaussian\nRTT ZC Rayleigh\nRTT ZC Log Normal\nRTT ZC Two Rayleigh\n\nTriangular Peak (s)\nTriangular Base (s)\nGaussian Peak (s)\nGaussian Base (s)\nRayleigh Peak (s)\nRayleigh Base (s)\nLog Normal Peak (s)\nLog Normal Base (s)\nTwo Rayleigh Peak (s)\nTwo Rayleigh Base (s)"
  # "Load the Database file in CSV format\nProvide the folder location only, \nand choose the CSV file from the drop down list"
  n1 = List Folder(path="Param Folder Path", pattern="*csv") -> (path out=w76:path, filenames=w39:string[], error out=w42:errorcluster)  [unwired: 2 in, 1 out]
  n2 = List Folder(path="Folder  Path", pattern="*csv") -> (path out=w75:path, filenames=w46:string[], error out=w47:errorcluster)  [unwired: 2 in, 1 out]
  n3 = List Folder(path="Folder  Path", pattern="*csv") -> (path out=w71:path, filenames=w56:string[], error out=w57:errorcluster)  [unwired: 2 in, 1 out]
  n4 = List Folder(path="Folder  Path", pattern="*csv") -> (path out=w72:path, filenames=w49:string[], error out=w52:errorcluster)  [unwired: 2 in, 1 out]
  n5 = List Folder(path="Folder  Path", pattern="*csv") -> (path out=w68:path, filenames=w61:string[], error out=w59:errorcluster)  [unwired: 2 in, 1 out]
  n6 = property on="FileName PPG" class="CmbBox"(error in=w47, "Strings[]"=w46) -> (error out=w45:errorcluster)  [unwired: 1 in, 1 out]
  n7 = property on="FileName P" class="CmbBox"(error in=w59, "Strings[]"=w61) -> (error out=w62:errorcluster)  [unwired: 1 in, 1 out]
  n8 = property on="FileName A" class="CmbBox"(error in=w57, "Strings[]"=w56) -> (error out=w55:errorcluster)  [unwired: 1 in, 1 out]
  n9 = property on="FileName U" class="CmbBox"(error in=w52, "Strings[]"=w49) -> (error out=w51:errorcluster)  [unwired: 1 in, 1 out]
  n10 = property on="FileName Param" class="CmbBox"(error in=w42, "Strings[]"=w39) -> (error out=w41:errorcluster)  [unwired: 1 in, 1 out]
  n11 = property on="FileName P" class="CmbBox"(error in=w62) -> (error out=w58:errorcluster, "Value"=w60:string)  [unwired: 1 in, 1 out]
  n12 = property on="FileName A" class="CmbBox"(error in=w55) -> (error out=w53:errorcluster, "Value"=w54:string)  [unwired: 1 in, 1 out]
  n13 = property on="FileName PPG" class="CmbBox"(error in=w45) -> (error out=w44:errorcluster, "Value"=w43:string)  [unwired: 1 in, 1 out]
  n14 = property on="FileName U" class="CmbBox"(error in=w51) -> (error out=w50:errorcluster, "Value"=w48:string)  [unwired: 1 in, 1 out]
  n15 = property on="FileName Param" class="CmbBox"(error in=w41) -> (error out=w40:errorcluster, "Value"=w38:string)  [unwired: 1 in, 1 out]
  n16 = Build Path(base path=w68, name or relative path=w60) -> (appended path=w69:path)
  n17 = Build Path(base path=w76, name or relative path=w38) -> (appended path=w77:path)
  n18 = Build Path(base path=w75, name or relative path=w43) -> (appended path=w74:path)
  n19 = Build Path(base path=w71, name or relative path=w54) -> (appended path=w70:path)
  n20 = Build Path(base path=w72, name or relative path=w48) -> (appended path=w73:path)
  n21 = call-poly <vilib>:"Read Delimited Spreadsheet.vi"("file path (dialog if empty)"=w77, "error in (no error)"=w40, "delimiter (\\t)"="," ("delimiter (\\t)")) -> ("all rows"=w63:dbl[][])  [unwired: 7 in, 5 out]
  n22 = call-poly <vilib>:"Read Delimited Spreadsheet.vi"("file path (dialog if empty)"=w74, "error in (no error)"=w44, "delimiter (\\t)"="," ("delimiter (\\t)")) -> ("all rows"=w64:dbl[][])  [unwired: 7 in, 5 out]
  n23 = call-poly <vilib>:"Read Delimited Spreadsheet.vi"("file path (dialog if empty)"=w70, "error in (no error)"=w53, "delimiter (\\t)"="," ("delimiter (\\t)")) -> ("all rows"=w66:dbl[][])  [unwired: 7 in, 5 out]
  n24 = call-poly <vilib>:"Read Delimited Spreadsheet.vi"("file path (dialog if empty)"=w73, "error in (no error)"=w50, "delimiter (\\t)"="," ("delimiter (\\t)")) -> ("all rows"=w65:dbl[][])  [unwired: 7 in, 5 out]
  n25 = call-poly <vilib>:"Read Delimited Spreadsheet.vi"("file path (dialog if empty)"=w69, "error in (no error)"=w58, "delimiter (\\t)"="," ("delimiter (\\t)")) -> ("all rows"=w67:dbl[][])  [unwired: 7 in, 5 out]
  n26 = while {
    tunnel: w67 -> [w290]
    tunnel: w66 -> [w291]
    tunnel: w65 -> [w289]
    tunnel: w64 -> [w265]
    tunnel: w63 -> [w288]
    shift-right: [w278] -> _
    shift-left: _ -> [w277]
    shift-left: _ -> [w276]
    tunnel: [w124] -> w31 mode=indexing
    tunnel: [w123] -> w30 mode=indexing
    tunnel: [w122] -> w35 mode=indexing
    tunnel: [w121] -> w34 mode=indexing
    tunnel: [w114] -> w24 mode=indexing
    tunnel: [w111] -> w22 mode=indexing
    tunnel: [w110] -> w21 mode=indexing
    tunnel: [w108] -> w15 mode=indexing
    tunnel: [w109] -> w18 mode=indexing
    tunnel: [w108] -> _
    tunnel: [w105] -> w7 mode=indexing
    tunnel: [w104] -> w14 mode=indexing
    tunnel: [w103] -> w6 mode=indexing
    tunnel: [w98] -> w1 mode=indexing
    i -> [w292]
    stop <- w280 stop-if-true
    # "Type, AIx"
    # "Golay Filter Fiducial Points"
    # "Butterworth Filter Fiducial Points"
    # "ID"
    # "PPG"
    # "Flow Velocity"
    # "Area"
    # "Pressure"
    # "Keep Last Sub ID as 0 to Stay at the saem Sub ID"
    n27 = Subtract(x=w277, y=w276) -> (x-y=→"Loop time (ms)":u32)
    n28 = case shown="False" "Loop Condition" {
      tunnel: "Start Subject ID" -> [w295 w298]
      tunnel: w292 -> [_ w297]
      tunnel: [w295 w296] -> w268
      frame False {
      }
      frame True {
        n29 = Add(x=w298, y=w297) -> (x+y=w296:i32)
      }
    }
    "Current ID" <- w268
    n30 = Equal?(x="Last Sub ID", y=w268) -> (x = y?=w280:bool)
    n31 = Wait (ms)(milliseconds to wait="Loop Wait Time (ms)") -> ()  [unwired: 1 out]
    n32 = flat-sequence {
      tunnel: w268 -> [w305]
      tunnel: w291 -> [w309]
      tunnel: w290 -> [w310]
      tunnel: w289 -> [w308]
      tunnel: w265 -> [w307]
      tunnel: w288 -> [w306]
      tunnel: [w304] -> w287
      tunnel: ["Original Sampling Rate (Hz)"] -> w286
      tunnel: [w302] -> w285
      tunnel: [w301] -> w284
      tunnel: [w300] -> w283
      tunnel: [w299] -> w282
      tunnel: w287 -> [w377]
      tunnel: w286 -> [w390]
      tunnel: w285 -> [w389]
      tunnel: w284 -> [w388]
      tunnel: w283 -> [w387]
      tunnel: w282 -> [w386]
      tunnel: [w377] -> w274
      tunnel: [w353] -> w273
      tunnel: [w487] -> w267
      tunnel: [w427] -> w266
      tunnel: w273 -> [w438]
      tunnel: w274 -> [w530]
      tunnel: [w438] -> w264
      tunnel: [w443] -> w263
      tunnel: [w481] -> w262
      tunnel: [w480] -> w261
      tunnel: [w479] -> w249
      tunnel: [w478] -> w248
      tunnel: [w469] -> w247
      tunnel: [w455] -> w125
      tunnel: [w452] -> w120
      tunnel: [w439] -> w119
      tunnel: [w446] -> w118
      tunnel: [w442] -> w117
      tunnel: [w441] -> w116
      tunnel: [w440] -> w115
      tunnel: [w428] -> w107
      tunnel: [w427] -> w102
      tunnel: [w411] -> w101
      tunnel: [w410] -> w100
      tunnel: [w409] -> w97
      tunnel: w266 -> [w663]
      tunnel: w267 -> [w664]
      tunnel: w264 -> [w630]
      tunnel: w263 -> [w656]
      tunnel: w262 -> [w657]
      tunnel: w261 -> [w633]
      tunnel: [w664] -> w260
      tunnel: [w663] -> w259
      tunnel: [w634] -> w258
      tunnel: [w629] -> w257
      tunnel: [w622] -> w256
      tunnel: [w620] -> w255
      tunnel: [w627] -> w254
      tunnel: [w628] -> w253
      tunnel: [w625] -> w252
      tunnel: [w621] -> w251
      tunnel: [w616] -> w250
      tunnel: w249 -> [w613]
      tunnel: w248 -> [w615]
      tunnel: w247 -> [w614]
      tunnel: [w615] -> w246
      tunnel: [w614] -> w245
      tunnel: [w613] -> w244
      tunnel: w125 -> [w611]
      tunnel: w120 -> [w658]
      tunnel: w119 -> [w610]
      tunnel: w118 -> [_]
      tunnel: w117 -> [w599]
      tunnel: w116 -> [w600]
      tunnel: w115 -> [w609]
      tunnel: [w608] -> w113
      tunnel: w107 -> [w607]
      tunnel: [w607] -> w106
      tunnel: w102 -> [w606]
      tunnel: w101 -> [w598]
      tunnel: w100 -> [w596]
      tunnel: [w596] -> w99
      tunnel: w97 -> [w595]
      tunnel: [w595] -> w96
      tunnel: [w991] -> w228
      tunnel: [w992] -> w229
      tunnel: w260 -> [w992]
      tunnel: w259 -> [w991]
      tunnel: w258 -> [w983]
      tunnel: w257 -> [w899]
      tunnel: w256 -> [w982]
      tunnel: w255 -> [w949]
      tunnel: w254 -> [w898]
      tunnel: w253 -> [w948]
      tunnel: w252 -> [w947]
      tunnel: w251 -> [w946]
      tunnel: [w927] -> w201
      tunnel: [w926] -> w183
      tunnel: [w913] -> w168
      tunnel: w250 -> [w911]
      tunnel: w246 -> [w910]
      tunnel: w245 -> [w909]
      tunnel: w244 -> [w912]
      tunnel: [w912] -> _
      tunnel: [w911] -> w152
      tunnel: [w910] -> w153
      tunnel: [w909] -> w160
      tunnel: [w908] -> w207
      tunnel: [w907] -> w206
      tunnel: [w906] -> w205
      tunnel: [w905] -> w204
      tunnel: [w904] -> w203
      tunnel: [w903] -> w202
      tunnel: [w895] -> w114
      tunnel: w113 -> [w894]
      tunnel: [w894] -> w112
      tunnel: [w893] -> w108
      tunnel: [w892] -> w109
      tunnel: w106 -> [w891]
      tunnel: [w891] -> w105
      tunnel: w99 -> [w890]
      tunnel: [w890] -> w98
      tunnel: w96 -> [w889]
      tunnel: [w889] -> w95
      frame #0 {
        # "Removal on NaN values"
        n33 = Index Array(array=w306, index (row)=w305) -> (element=w332:dbl[])  [unwired: 1 in]
        n34 = Index Array(array=w309, index (row)=w305) -> (element=w318:dbl[])  [unwired: 1 in]
        n35 = Index Array(array=w308, index (row)=w305) -> (element=w321:dbl[])  [unwired: 1 in]
        n36 = Index Array(array=w307, index (row)=w305) -> (element=w322:dbl[])  [unwired: 1 in]
        n37 = Index Array(array=w310, index (row)=w305) -> (element=w317:dbl[])  [unwired: 1 in]
        n38 = Array Size(array=w322) -> (size(s)=w323:i32)
        n39 = Array Size(array=w318) -> (size(s)=w319:i32)
        n40 = Array Size(array=w317) -> (size(s)=w316:i32)
        n41 = Array Size(array=w321) -> (size(s)=w320:i32)
        n42 = Array Size(array=w332) -> (size(s)=w333:i32)
        n43 = Array Subset(array=w318, index=1, length=w319) -> (w326:dbl[])
        n44 = Array Subset(array=w321, index=1, length=w320) -> (w328:dbl[])
        n45 = Array Subset(array=w322, index=1, length=w323) -> (w330:dbl[])
        n46 = Array Subset(array=w317, index=1, length=w316) -> (w324:dbl[])
        n47 = Array Subset(array=w332, index=1, length=w333) -> (w334:dbl[])
        n48 = To Double Precision Float(number=w328) -> (double precision float=w329:dbl[])
        n49 = To Double Precision Float(number=w330) -> (double precision float=w331:dbl[])
        n50 = To Double Precision Float(number=w326) -> (double precision float=w327:dbl[])
        n51 = To Double Precision Float(number=w324) -> (double precision float=w325:dbl[])
        n52 = To Double Precision Float(number=w334) -> (double precision float=w304:dbl[])
        n53 = for {
          tunnel: w331 -> [w337] mode=indexing
          tunnel: [w337] -> w302 mode=indexing if=w335
          n54 = Not A Number/Path/Refnum?(number/path/refnum=w337) -> (NaN/Path/Refnum?=w336:bool)
          n55 = Not(x=w336) -> (.not. x?=w335:bool)
        }
        n56 = for {
          tunnel: w325 -> [w346] mode=indexing
          tunnel: [w346] -> w301 mode=indexing if=w344
          n57 = Not A Number/Path/Refnum?(number/path/refnum=w346) -> (NaN/Path/Refnum?=w345:bool)
          n58 = Not(x=w345) -> (.not. x?=w344:bool)
        }
        n59 = for {
          tunnel: w327 -> [w343] mode=indexing
          tunnel: [w343] -> w300 mode=indexing if=w341
          n60 = Not A Number/Path/Refnum?(number/path/refnum=w343) -> (NaN/Path/Refnum?=w342:bool)
          n61 = Not(x=w342) -> (.not. x?=w341:bool)
        }
        n62 = for {
          tunnel: w329 -> [w340] mode=indexing
          tunnel: [w340] -> w299 mode=indexing if=w338
          n63 = Not A Number/Path/Refnum?(number/path/refnum=w340) -> (NaN/Path/Refnum?=w339:bool)
          n64 = Not(x=w339) -> (.not. x?=w338:bool)
        }
      }
      frame #1 {
        # "Area to Diameter"
        # "m^3 to mm^3"
        # "m^3/s = 1000 l/s = 1M ml/s"
        # "Removal of Baseline Wandering"
        # "Ensuring Cycle is from Minima to Minima"
        # "Re-Sample"
        n65 = Reciprocal(x=w390) -> (1/x=w391:dbl)
        n66 = case shown="True" "Re Sample?" {
          tunnel: w391 -> [w397 w404]
          tunnel: [w395 w408] -> w370
          tunnel: [w397 w398] -> w362
          tunnel: [w396 w407] -> w365
          tunnel: [w394 w406] -> w371
          tunnel: [w393 w405] -> w378
          tunnel: w388 -> [w395 w402]
          tunnel: w387 -> [w396 w401]
          tunnel: w386 -> [w394 w400]
          tunnel: w389 -> [w393 w399]
          frame False {
          }
          frame True {
            n67 = call "Re-Sample Waveform (SubVI).vi"("Filtered w/f"=w399, "old dt"=w404, "Re Sample Rate(Hz)"="Re Sample Rate(Hz)") -> ("Re-sampled w/f"=w405:dbl[])  [unwired: 7 in, 1 out]
            n68 = call "Re-Sample Waveform (SubVI).vi"("Filtered w/f"=w402, "old dt"=w404, "Re Sample Rate(Hz)"="Re Sample Rate(Hz)") -> ("Re-sampled w/f"=w408:dbl[], "new dt"=w398:dbl)  [unwired: 7 in]
            n69 = call "Re-Sample Waveform (SubVI).vi"("Filtered w/f"=w401, "old dt"=w404, "Re Sample Rate(Hz)"="Re Sample Rate(Hz)") -> ("Re-sampled w/f"=w407:dbl[])  [unwired: 7 in, 1 out]
            n70 = call "Re-Sample Waveform (SubVI).vi"("Filtered w/f"=w400, "old dt"=w404, "Re Sample Rate(Hz)"="Re Sample Rate(Hz)") -> ("Re-sampled w/f"=w406:dbl[])  [unwired: 7 in, 1 out]
          }
        }
        "dt" <- w362
        n71 = Multiply(x=w365, y=w371) -> (x*y=w368:dbl[])
        n72 = Divide(x=4.0, y=3.141592653589793) -> (x/y=w383:dbl)
        n73 = Multiply(x=w383, y=w365) -> (x*y=w384:dbl[])
        n74 = Square Root(x=w384) -> (sqrt(x)=w385:dbl[])
        n75 = Multiply(x=w385, y=1000.0) -> (x*y=w379:dbl[])
        n76 = Multiply(x=1000000.0, y=w365) -> (x*y=w363:dbl[])
        n77 = Multiply(x=w368, y=1000000.0) -> (x*y=w366:dbl[])
        n78 = call "Minima_to_Minima (SubVI).vi"("Y"=w370) -> ("length"=w360:dbl, "index"=w361:i32, "Array"=w369:dbl[])  [unwired: 8 in]
        n79 = Array Subset(array=w363, index=w361, length=w360) -> (w351:dbl[])
        n80 = Array Subset(array=w366, index=w361, length=w360) -> (w348:dbl[])
        n81 = Array Subset(array=w371, index=w361, length=w360) -> (w349:dbl[])
        n82 = Array Subset(array=w379, index=w361, length=w360) -> (w374:dbl[])
        n83 = Array Subset(array=w378, index=w361, length=w360) -> (w372:dbl[])
        n84 = call "Baseline_basic (SubVI).vi"("S/g with baseline drift"=w369) -> ("Corrected"=w376:dbl[])  [unwired: 10 in]
        n85 = call "Baseline_basic (SubVI).vi"("S/g with baseline drift"=w351) -> ("Corrected"=w350:dbl[])  [unwired: 10 in]
        n86 = call "Baseline_basic (SubVI).vi"("S/g with baseline drift"=w348) -> ()  [unwired: 10 in, 1 out]
        n87 = call "Baseline_basic (SubVI).vi"("S/g with baseline drift"=w374) -> ("Corrected"=w375:dbl[])  [unwired: 10 in]
        n88 = call "Baseline_basic (SubVI).vi"("S/g with baseline drift"=w349) -> ("Corrected"=w347:dbl[])  [unwired: 10 in]
        n89 = call "Baseline_basic (SubVI).vi"("S/g with baseline drift"=w372) -> ("Corrected"=w373:dbl[])  [unwired: 10 in]
        n90 = Bundle By Name("dt"=w362, "Y"=w376) -> (w359:waveform(dbl))  [unwired: 1 in]
        "Pressure" <- w359
        n91 = Bundle By Name("dt"=w362, "Y"=w350) -> (w358:waveform(dbl))  [unwired: 1 in]
        "Area" <- w358
        n92 = Bundle By Name("dt"=w362, "Y"=w347) -> (w356:waveform(dbl))  [unwired: 1 in]
        "Flow Velocity" <- w356
        n93 = Bundle By Name("dt"=w362, "Y"=w375) -> (w357:waveform(dbl))  [unwired: 1 in]
        "Diameter" <- w357
        n94 = Bundle By Name("dt"=w362, "Y"=w373) -> (w355:waveform(dbl))  [unwired: 1 in]
        "PPG" <- w355
        n95 = Bundle By Name("dt"=w362, "Y"=w348) -> (w352:waveform(dbl))  [unwired: 1 in]
        "Flow Rate" <- w352
        n96 = Bundle By Name(cluster=T10 {"Pressure (mmHg)"={"t0"=timestamp(0 s since 1904-01-01), "dt"=0.002, "Y"=array[411 elements]}, "Area (mm^2)"={"t0"=timestamp(0 s since 1904-01-01), "dt"=0.002, "Y"=array[411 elements]}, "Flow Velocity (m/s)"={"t0"=timestamp(0 s since 1904-01-01), "dt"=0.002, "Y"=array[411 elements]}, "Flow Rate (ml/s)"={"t0"=timestamp(0 s since 1904-01-01), "dt"=0.002, "Y"=array[411 elements]}, "Diameter (mm)"={"t0"=timestamp(0 s since 1904-01-01), "dt"=0.002, "Y"=array[411 elements]}, "PPG"={"t0"=timestamp(0 s since 1904-01-01), "dt"=0.002, "Y"=array[411 elements]}} ("input cluster"), "Pressure (mmHg)"=w359, "Area (mm^2)"=w358, "Diameter (mm)"=w357, "Flow Velocity (m/s)"=w356, "Flow Rate (ml/s)"=w352, "PPG"=w355) -> (w353:T10)
        "Hemodynamic Param" <- w377
      }
      frame #2 {
        w489 = 1000.0 ("threshold y")
        w508 = TRUE ("Derivative filter on?")
        # "LS Peak Type C"
        # "LS Peak Type A"
        # "Calcilaion of Stiffness Markers"
        n97 = Unbundle By Name(w438) -> ("Flow Rate (ml/s)"=w437:waveform(dbl))
        n98 = Unbundle By Name(w438) -> ("Pressure (mmHg)"=w461:waveform(dbl), "Flow Rate (ml/s)"=w466:waveform(dbl))
        n99 = Unbundle By Name(w437) -> ("Y"=w436:dbl[], "dt"=w416:dbl)
        n100 = Unbundle By Name(w461) -> ("Y"=w509:dbl[], "dt"=w524:dbl)
        n101 = call <vilib>:"Peak Detector.vi"("X"=w436) -> ("Amplitudes"=w434:dbl[], "Locations"=w435:dbl[])  [unwired: 6 in, 3 out]
        n102 = Unbundle By Name(w438) -> ("Pressure (mmHg)"=w566:waveform(dbl), "Flow Rate (ml/s)"=w565:waveform(dbl))
        n103 = call "Peaks select ( SubVI).vi"("Locations"=w435, "Amplitude"=w434, "No of peaks Required"=2, "Min seperation B/W peaks"=10.0) -> ("Locations"=w417:dbl[], "Amplitude"=w431:dbl[])  [unwired: 3 in, 1 out]
        "Amplitude" <- w431
        n104 = call "Derivative PCA Cycles (SubVI).vi"("Derivative filter on?"=w508, "Derivative LPF cutoff (Hz)"="Derivative LPF cutoff (Hz)", "dt"=w524, "Waveform (samples) in"=w509) -> ("AIx Related"=w427:T9, "Fid. Points (SDW)"=w487:T4)  [unwired: 5 in, 1 out]
        "AIx" <- w427
        "Fid. Points (SDW)" <- w487
        n105 = call "SG Derivatives (SubVI).vi"("SG Filter Config"="SG Filter Config", "dt"=w524, "Pre. Cycle"=w509) -> ("Fid. Points"=w409:T12, "waveforms"=w526:T13)  [unwired: 6 in, 1 out]
        n106 = Unbundle By Name(w466) -> ("dt"=w447:dbl, "Y"=w515:dbl[])
        n107 = call "Derivative LFR cycles (SubVI).vi"("Derivative LPF cutoff (Hz)"="Derivative LPF cutoff (Hz)", "Derivative filter on?"=w508, "dt"=w447, "Waveform (samples) in"=w509) -> ("Fourth derivative (samples)"=w467:dbl[], "Second derivative (samples)"=w468:dbl[], "First derivative (samples)"=w465:dbl[], "Waveform (samples) out"=w450:dbl[])  [unwired: 4 in]
        n108 = Index Array(array=w431) -> (element #1=w430:dbl, element #2=w429:dbl)  [unwired: 2 in]
        n109 = Multiply(x=w417, y=w416) -> (x*y=w415:dbl[])
        n110 = Divide(x=w429, y=w430) -> (x/y=w428:dbl)
        "A1/A2" <- w428
        n111 = Bundle By Name(cluster=w461, "Y"=w465) -> (w464:waveform(dbl))
        n112 = Bundle By Name(cluster=w461, "Y"=w468) -> (w463:waveform(dbl))
        n113 = Index Array(array=w415) -> (element #1=w414:dbl, element #2=w413:dbl)  [unwired: 2 in]
        n114 = Bundle By Name(cluster=w461, "Y"=w467) -> (w462:waveform(dbl))
        n115 = Array Max & Min(array=w515) -> (max index (indices)=w514:i32)  [unwired: 3 out]
        n116 = call "Input Impedence_Freq Domian(SubVI).vi"("Settings"="Settings", "Flow Rate (ml/s)"=w565, "Pressure (mmHg)"=w566) -> ("Zo (at 0 Hz) (mmHg/ml/s)"=→"PVR (mmHg/ml/s)":dbl, "Zc (mmHg/ml/s)"=w594:dbl, "Zo - Phase Spectrum"=→"Input Impedence - Phase Spectrum":waveform(dbl), "Zo - Magnitude Spectrum"=→"Input Impedence - Magnitude Spectrum":waveform(dbl))  [unwired: 5 in]
        "Zc (mmHg/ml/s)" <- w594
        n117 = Unbundle By Name(w438) -> ("Pressure (mmHg)"=w552:waveform(dbl), "Diameter (mm)"=w551:waveform(dbl))
        n118 = Unbundle By Name(w438) -> ("Pressure (mmHg)"=w559:waveform(dbl), "Flow Velocity (m/s)"=w558:waveform(dbl), "Area (mm^2)"=w561:waveform(dbl))
        n119 = Unbundle By Name(w438) -> ("Pressure (mmHg)"=w529:waveform(dbl), "Diameter (mm)"=w528:waveform(dbl))
        n120 = Unbundle By Name(w526) -> ("FDW"=w523:waveform(dbl), "SDW"=w522:waveform(dbl), "FoDW"=w426:waveform(dbl))
        n121 = Multiply(x=w447, y=w514) -> (x*y=w452:dbl)
        "True Flow Peak (sec)" <- w452
        n122 = Unbundle(w487) -> ("SF"=w521:dbl, "ER"=w519:dbl, "IP"=w518:dbl, "DN"=w517:dbl, "SDW ZC 1"=w520:dbl, "MX"=w504:dbl, "FDW ZC"=w505:dbl, "FoDW ZC"=w506:dbl)  [unwired: 1 out]
        n123 = Build Array(w521, w519, w518, w517, w520, w504, w505, w506, w452) -> (w513:dbl[])
        n124 = Index Array(array=w530, index #1=17 ("index"), index #6=2 ("index"), index #8=0 ("index")) -> (element #1=w470:dbl, element #2=w471:dbl, element #3=w472:dbl, element #4=w473:dbl, element #5=w474:dbl, element #6=w475:dbl, element #7=w476:dbl, element #8=w477:dbl)  [unwired: 5 in]
        "AP (mmHg)" <- w470
        "AIx (%)" <- w471
        "Tr (ms)" <- w472
        "Aortic PWV (m/s)" <- w473
        "cf-PWV (m/s)" <- w474
        "SV (ml)" <- w475
        "CO (l/min)" <- w476
        "Age (years)" <- w477
        n125 = Unbundle By Name(w528) -> ("Y"=w534:dbl[])
        n126 = Unbundle By Name(w426) -> ("dt"=w422:dbl, "Y"=w425:dbl[])
        n127 = Unbundle By Name(w559) -> ("Y"=w557:dbl[])
        n128 = Unbundle By Name(w558) -> ("Y"=w556:dbl[])
        n129 = Unbundle By Name(w529) -> ("Y"=w542:dbl[])
        n130 = call "Min_Max_Amp (SubVI).vi"("waveform"=w561) -> ("MN"=w502:dbl)  [unwired: 8 in, 2 out]
        n131 = Unbundle By Name(w552) -> ("Y"=w554:dbl[])
        n132 = Unbundle By Name(w551) -> ("Y"=w553:dbl[])
        n133 = Divide(x=w513, y=w447) -> (x/y=w512:dbl[])
        n134 = Array Size(array=w534) -> (size(s)=w536:i32)
        n135 = Array Size(array=w542) -> (size(s)=w543:i32)
        n136 = Multiply(x=w452, y=1000.0 ("threshold y")) -> (x*y=w483:dbl)
        n137 = call <vilib>:"Peak Detector.vi"("X"=w425) -> ("Amplitudes"=w424:dbl[], "Locations"=w420:dbl[])  [unwired: 6 in, 3 out]
        n138 = Divide(x=w502, y=1000000.0) -> (x/y=w550:dbl)
        n139 = call "Pts_Plot (SubVI).vi"("Ref WF"=w509, "Locations"=w512) -> ("Waveform"=w516:dbl[])  [unwired: 9 in]
        n140 = call "PWV_BH(SubVI).vi"("Diameter (mm)"=w553, "Pressure (mmhg)"=w554) -> ("PWV (m/s) (BH approx.)"=w548:dbl)  [unwired: 7 in, 2 out]
        "PWV (BH) (m/s)" <- w548
        n141 = Unbundle By Name(w438) -> ("Pressure (mmHg)"=w591:waveform(dbl), "Flow Rate (ml/s)"=w588:waveform(dbl))
        n142 = call "PWV_dPdU(SubVI).vi"("Flow Velocity (m/s)"=w556, "Pressure (mmHg)"=w557) -> ("PWV (m/s) (dPdU)"=w555:dbl)  [unwired: 9 in]
        "PWV (dPdU) (m/s)" <- w555
        n143 = Divide(x=w543, y=2.0 ("Min Value")) -> (x/y=w541:dbl)
        n144 = Divide(x=w536, y=2.0 ("Min Value")) -> (x/y=w537:dbl)
        n145 = Bundle By Name("Y"=w516, "dt"=w447) -> (w459:waveform(dbl))  [unwired: 1 in]
        n146 = Merge Signals(w461, w464, w463, w462, w466, w459) -> (→"Derivatives of P(t) 2":dynamicdata)
        n147 = Array Subset(array=w534, length=w537) -> (w538:dbl[])  [unwired: 1 in]
        n148 = call "Input Impedence_Time Domain(SubVI).vi"("Ad (m^2)"=w550, "PWV (m/s)"=w555) -> ("Zc (mmHg/ml/s)"=w592:dbl)  [unwired: 9 in]
        "Zc (mmHg/ml/s)" <- w592
        n149 = call "Input Impedence_Time Domain(SubVI).vi"("Ad (m^2)"=w550, "PWV (m/s)"=w548) -> ("Zc (mmHg/ml/s)"=→"Zc (mmHg/ml/s)":dbl)  [unwired: 9 in]
        n150 = Array Subset(array=w542, length=w541) -> (w540:dbl[])  [unwired: 1 in]
        n151 = Build Array(w477, w476, w475, w474, w473, w472, w471, w470) -> (w469:dbl[])
        n152 = call "Peaks select ( SubVI).vi"("Locations"=w420, "Amplitude"=w424, "No of peaks Required"=10, "Min seperation B/W peaks"="Min seperation B/W peaks") -> ("Locations"=w419:dbl[])  [unwired: 3 in, 2 out]
        n153 = Unbundle By Name(w487) -> ("SDW ZC 2"=w411:dbl, "IP"=w457:dbl, "SDW ZC 1"=w412:dbl, "DN"=w443:dbl, "MX"=w444:dbl, "FoDW ZC"=w456:dbl)
        "T_Ejection Period (sec)" <- w443
        n154 = Unbundle By Name(w409) -> ("SD ZC 1 (s)"=w497:dbl)
        n155 = Array Max & Min(array=w538) -> (max value=w539:dbl, min value=w532:dbl)  [unwired: 2 out]
        n156 = Array Max & Min(array=w540) -> (max value=w500:dbl, min value=w499:dbl)  [unwired: 2 out]
        "SBP (mmHg)" <- w500
        "DBP (mmHg)" <- w499
        n157 = Merge Signals(w461, w523, w522, w426, w466, w459) -> (→"Derivatives of P(t)":dynamicdata)
        n158 = Array Size(array=w450) -> (size(s)=w449:i32)
        n159 = Multiply(x=w422, y=w419) -> (x*y=w418:dbl[])
        "Peak of FoDW" <- w418
        n160 = Subtract(x=w539, y=w532) -> (x-y=w531:dbl)
        n161 = Subtract(x=w449, y=1) -> (x-y=w445:i32)
        n162 = call "Classical WSA (SubVI).vi"("Zc (mmHg/ml/s)"=w594, "Flow Rate (ml/s)"=w588, "Pressure (mmHg)"=w591) -> ("WSA Waveforms"=w569:T14)  [unwired: 8 in]
        n163 = call "Classical WSA (SubVI).vi"("Zc (mmHg/ml/s)"=w592, "Flow Rate (ml/s)"=w588, "Pressure (mmHg)"=w591) -> ("WSA Waveforms"=w568:T14)  [unwired: 8 in]
        n164 = for {
          tunnel: w418 -> [_] mode=indexing
        }
        n165 = Unbundle By Name(w438) -> ("Pressure (mmHg)"=w486:waveform(dbl), "Flow Rate (ml/s)"=w482:waveform(dbl))
        n166 = call "Stiffness (SubVI).vi"("C_DBP"=w499, "C_SBP"=w500, "dD"=w531, "Dd"=w532) -> ("Beta"=w545:dbl, "Ep"=w546:dbl, "AC"=w501:dbl, "PWV_b"=w547:dbl)  [unwired: 3 in]
        "Beta" <- w545
        "Ep" <- w546
        "AC" <- w501
        "PWV (BH)" <- w547
        n167 = Multiply(x=w447, y=w445) -> (x*y=w440:dbl)
        n168 = Unbundle By Name(w569) -> ("P FWD"=w567:waveform(dbl), "P BWD"=w586:waveform(dbl), "Q FWD"=w585:waveform(dbl), "Q BWD"=w584:waveform(dbl))
        n169 = Unbundle By Name(w568) -> ("P FWD"=w573:waveform(dbl), "P BWD"=w572:waveform(dbl))
        n170 = Unbundle By Name(w568) -> ("P FWD"=w583:waveform(dbl), "P BWD"=w582:waveform(dbl), "Q FWD"=w581:waveform(dbl), "Q BWD"=w580:waveform(dbl))
        n171 = Unbundle By Name(w569) -> ("P FWD"=w571:waveform(dbl), "P BWD"=w570:waveform(dbl))
        n172 = Greater?(x=w412, y=w444) -> (0:w496:bool)
        n173 = Subtract(x=w440, y=w443) -> (x-y=w446:dbl)
        n174 = Greater?(x=w457, y=w452) -> (0:w458:bool)
        n175 = Select(t=w497, s=w496, f=w412) -> (s? t:f=w453:dbl)
        "T_Flow Peak (sec)" <- w453
        n176 = call "Min_Max_Amp (SubVI).vi"("waveform"=w482) -> ("MX"=w481:dbl)  [unwired: 8 in, 2 out]
        n177 = Unbundle By Name(w572) -> ("Y"=w576:dbl[])
        n178 = Unbundle By Name(w573) -> ("Y"=w577:dbl[])
        n179 = Unbundle By Name(w570) -> ("Y"=w574:dbl[])
        n180 = Unbundle By Name(w571) -> ("Y"=w575:dbl[])
        n181 = Select(t=w457, s=w458, f=w456) -> (s? t:f=w439:dbl)
        n182 = Merge Signals(w591, w567, w586) -> (→"WSA P - Freq. Domain":dynamicdata)
        n183 = Merge Signals(w588, w585, w584) -> (→"WSA Q - Freq. Domain":dynamicdata)
        n184 = Build Array(w545, w546, w501, w547, w500, w499) -> (w478:dbl[])
        n185 = Merge Signals(w591, w583, w582) -> (→"WSA P - Time. Domain":dynamicdata)
        n186 = Merge Signals(w588, w581, w580) -> (→"WSA Q - Time Domain":dynamicdata)
        n187 = Unbundle By Name(w486) -> ("dt"=w494:dbl, "Y"=w491:dbl[])
        n188 = Build Array(w453, w443) -> (w493:dbl[])
        n189 = Bundle By Name(cluster=T8 {"Flow Peak (sec)"=0.078, "Flow Peak (Amp)"=0.078} ("Actual Flow"), "Flow Peak (sec)"=w452, "Flow Peak (Amp)"=w481) -> (→"Reference Flow Rate":T8)
        n190 = call "Get RM_RI (SubVI).vi"("Bwd"=w576, "Fwd"=w577) -> ("Reflection Markers"=→"Reflection Markers\n(Time Domain WSA)":T15)  [unwired: 9 in]
        n191 = call "Get RM_RI (SubVI).vi"("Bwd"=w574, "Fwd"=w575) -> ("Reflection Markers"=→"Reflection Markers\n(Freq. Domain WSA)":T15)  [unwired: 9 in]
        n192 = Less?(x=w439, y=w444) -> (x < y?=w455:bool)
        n193 = Divide(x=w493, y=w494) -> (x/y=w495:dbl[])
        n194 = Build Array(w439, w444) -> (w451:dbl[])
        n195 = Multiply(x=w453, y=w489) -> (x*y=w485:dbl)
        n196 = Multiply(x=w443, y=w489) -> (x*y=w498:dbl)
        n197 = call "Pts_Plot (SubVI).vi"("Ref WF"=w491, "Locations"=w495) -> ("Waveform"=w492:dbl[])  [unwired: 9 in]
        n198 = call-poly <vilib>:"Mean.vi"("X"=w451) -> ("mean"=w442:dbl)  [unwired: 1 out]
        n199 = Build Array(w439, w443) -> (w454:dbl[])
        n200 = Bundle By Name("dt"=w494, "Y"=w492) -> (w480:waveform(dbl))  [unwired: 1 in]
        n201 = Build Array(w483, w485, w498, w481) -> (w479:dbl[])
        n202 = call-poly <vilib>:"Mean.vi"("X"=w454) -> ("mean"=w441:dbl)  [unwired: 1 out]
        n203 = Build Array(w414, w413, w412, w411) -> (w410:dbl[])
      }
      frame #3 {
        w623 = 1000000.0
        w639 = 20 ("length")
        # "LS Peak Type C"
        # "LS Peak Type A"
        # "IP < MX ---> Type A  or B"
        # "Flow Amp"
        # "IP"
        # "Pressure"
        # "Reference Flow"
        # "m-Rayeligh Flow"
        # "Triangular Flow"
        # "Multi-Rayleigh Flow Rate Model"
        # "T_Ejection Period (s)"
        # "T_Flow Peak (s)"
        n204 = Unbundle By Name(w606) -> ("AIx (%) (4th D ZC)"=w605:dbl)
        n205 = Unbundle By Name(w630) -> ("Pressure (mmHg)"=w659:waveform(dbl), "Flow Rate (ml/s)"=w661:waveform(dbl))
        n206 = Multiply(x=w605, y=0.0033 ("T_Flow Start (s)")) -> (x*y=w603:dbl)
        n207 = Add(x=w603, y=0.4006 ("T_Flow Start (s)")) -> (x+y=→"A2/A1":dbl)
        n208 = while {
          shift-right: [w692] -> w634
          shift-left: w659 -> [w693]
          shift-right: [w690] -> w629
          shift-left: w661 -> [w691]
          shift-right: [w686] -> _
          shift-left: w658 -> [w689]
          shift-right: [w685] -> _
          shift-left: w656 -> [w688]
          shift-right: [w684] -> _
          shift-left: w657 -> [w687]
          shift-right: [w682] -> _
          shift-left: T11."1-Rayleigh Model" ("Enum") -> [w683]
          shift-right: [w677] -> w618
          shift-left: _ -> [w675]
          shift-right: [w678] -> w617
          shift-left: _ -> [w674]
          shift-right: [w680] -> w627
          shift-left: _ -> [w673]
          shift-right: [w676] -> w619
          shift-left: _ -> [w672]
          shift-right: [w679] -> w608
          shift-left: _ -> [w671]
          tunnel: w611 -> [w670]
          tunnel: w610 -> [w669]
          tunnel: w598 -> [w668]
          tunnel: w598 -> [w667]
          tunnel: w609 -> [w666]
          tunnel: "A2/A1 2" -> [w665]
          stop <- w681 stop-if-true
          n209 = case shown="\"5-Rayleigh Model\"" w683 {
            tunnel: [w699 w734 w811 w836 w861 w882] -> w692
            tunnel: w693 -> [w699 w734 w811 w836 w861 w882]
            tunnel: [w712 w723 w818 w843 w866 w881] -> w690
            tunnel: w691 -> [w712 w723 w818 w843 w866 w881]
            tunnel: w689 -> [w697 w729 w809 w834 w859 w880]
            tunnel: w688 -> [w698 w728 w810 w835 w860 w879]
            tunnel: w687 -> [w694 w732 w807 w832 w856 w878]
            tunnel: [w697 w729 w809 w834 w859 w880] -> w686
            tunnel: [w698 w728 w810 w835 w860 w879] -> w685
            tunnel: [w694 w732 w807 w832 w856 w878] -> w684
            tunnel: [w702 w737 w814 w839 T11."STOP" ("Enum") _] -> w682
            tunnel: [_ _ _ _ _ TRUE] -> w681
            tunnel: [w700 w726 w812 w837 w862 w886] -> w680
            tunnel: [w705 w740 w816 w841 w864 w884] -> w679
            tunnel: [w695 w724 w806 w831 w857 w887] -> w678
            tunnel: [w704 w738 w817 w842 w865 w888] -> w677
            tunnel: [1.0 ("T_Flow Start (s)") 2.0 ("T_Flow Start (s)") 3.0 ("T_Flow Start (s)") 4.0 ("T_Flow Start (s)") 5.0 ("T_Flow Start (s)") w885] -> w676
            tunnel: w675 -> [_ _ _ _ _ w888]
            tunnel: w674 -> [_ _ _ _ _ w887]
            tunnel: w673 -> [_ _ _ _ _ w886]
            tunnel: w672 -> [_ _ _ _ _ w885]
            tunnel: w671 -> [_ _ _ _ _ w884]
            tunnel: w670 -> [_ w735 _ _ _ _]
            tunnel: w669 -> [_ w721 _ _ _ _]
            tunnel: w668 -> [_ w733 _ _ _ _]
            tunnel: w667 -> [_ w725 _ _ _ _]
            tunnel: w666 -> [_ w722 _ _ _ _]
            tunnel: w665 -> [_ w719 _ _ _ _]
            frame "1-Rayleigh Model" {
              (unwired) TRUE
              w696 = 0.0 ("T_Flow Start (s)")
              n210 = call "Get 1-Rayleigh Parameters (SubVI).vi"("Flow Peak Amp."=w694, "T_Flow Start (s)"=w696, "T_Flow Peak (s)"=w697, "T_Ejection period (s)"=w698, "Pressure (mmHg)"=w699) -> ("Optimised Parameter"=w695:dbl[])  [unwired: 6 in]
              n211 = call "N_Rayleigh_Flow Model (SubVI).vi"("PSQ (ml/s)"=w694, "T_Flow Start"=w696, "Parameters (1XN)"=w695, "Pressure (mmHg)"=w699) -> ("n-Rayleigh Model Flow"=w700:waveform(dbl))  [unwired: 4 in, 1 out]
              n212 = call "Peak_Base_Error_Check (SubVI).vi"("Model Flow"=w700, "T_Ejection Period (s)"=w698, "T_Flow Peak (s)"=w697) -> ("Error"=w715:dbl[])  [unwired: 5 in, 3 out]
              n213 = Unbundle By Name(w712) -> ("Y"=w713:dbl[])
              n214 = Unbundle By Name(w700) -> ("Y"=w714:dbl[])
              n215 = call "Error Analysis (SubVI).vi"("Measured Wave"=w714, "Reference Wave"=w713) -> ("RMSE"=w704:dbl)  [unwired: 6 in, 3 out]
              n216 = Multiply(x=w715, y=1000.0 ("T_Flow Start (s)")) -> (x*y=w705:dbl[])
              n217 = Index Array(array=w705) -> (element #1=w711:dbl, element #2=w710:dbl)  [unwired: 2 in]
              n218 = Less Or Equal?(x=w710, y=2.0 ("T_Flow Start (s)")) -> (x <= y?=w706:bool)
              n219 = Less Or Equal?(x=w711, y=1.0 ("T_Flow Start (s)")) -> (x <= y?=w707:bool)
              n220 = And(x=w707, y=w706) -> (x .and. y?=w701:bool)
              n221 = case shown="False" w701 {
                tunnel: [T11."2-Rayleigh Model" ("Enum") T11."STOP" ("Enum")] -> w702
                frame False {
                }
                frame True {
                }
              }
            }
            frame "2-Rayleigh Model" {
              n222 = case shown="True" w735 {
                tunnel: w734 -> [w758 w785]
                tunnel: w728 -> [w766 w784]
                tunnel: w729 -> [w768 w787]
                tunnel: w733 -> [_ w783]
                tunnel: w732 -> [w775 w801]
                tunnel: [w754 w791] -> w731
                tunnel: [w759 w789] -> w730
                tunnel: [w774 w796] -> w726
                tunnel: [w773 w799] -> w727
                tunnel: w725 -> [w765 _]
                tunnel: [w772 w798] -> w724
                tunnel: w723 -> [w771 _]
                tunnel: w722 -> [_ _]
                tunnel: w721 -> [w756 w782]
                tunnel: [w763 w792] -> w720
                tunnel: w719 -> [w755 w778]
                frame False {
                  w751 = 1.0 ("T_Flow Start (s)")
                  # "LSP"
                  # "IP"
                  # "Type C"
                  n223 = call "Get 2-Rayleigh Parameters (SubVI).vi"("Flow Peak Amp."=w751, "T_Flow Start (s)"=0.0, "T_Flow Peak (s)"=w768, "T_Ejection period (s)"=w765, "Pressure (mmHg)"=w758) -> ("Optimised Parameter"=w757:dbl[])  [unwired: 6 in]
                  n224 = call "Get 2-Rayleigh Parameters (SubVI).vi"("Flow Peak Amp."=w755, "T_Flow Start (s)"=w756, "T_Flow Peak (s)"=w765, "T_Ejection period (s)"=w766, "Pressure (mmHg)"=w758) -> ("Optimised Parameter"=w761:dbl[])  [unwired: 6 in]
                  n225 = call "Get 1-Rayleigh Parameters (SubVI).vi"("Flow Peak Amp."=w755, "T_Flow Start (s)"=w756, "T_Flow Peak (s)"=w765, "T_Ejection period (s)"=w766, "Pressure (mmHg)"=w758) -> ()  [unwired: 6 in, 1 out]
                  n226 = Build Array (concatenate)(w757, w761) -> (w772:dbl[])
                  n227 = call "N_Rayleigh_Flow Model (SubVI).vi"("PSQ (ml/s)"=w751, "T_Flow Start"=0.0 ("T_Flow Start (s)"), "Parameters (1XN)"=w757, "Pressure (mmHg)"=w758) -> ("Waveform Graph"=w753:dbl[][], "n-Rayleigh Model Flow"=w754:waveform(dbl))  [unwired: 4 in]
                  n228 = call "N_Rayleigh_Flow Model (SubVI).vi"("PSQ (ml/s)"=w755, "T_Flow Start"=w756, "Parameters (1XN)"=w761, "Pressure (mmHg)"=w758) -> ("Waveform Graph"=w760:dbl[][], "n-Rayleigh Model Flow"=w759:waveform(dbl))  [unwired: 4 in]
                  n229 = Unbundle By Name(w754) -> ("Y"=w777:dbl[])
                  n230 = Unbundle By Name(w759) -> ("Y"=w762:dbl[])
                  n231 = Compound Arithmetic op=ADD(w777, w762) -> (w770:dbl[])
                  n232 = call "Scale_0_1 (SubVI).vi"("BLine D"=w770) -> ("Array"=w769:dbl[])  [unwired: 10 in]
                  n233 = Multiply(x=w775, y=w769) -> (x*y=w776:dbl[])
                  n234 = call "Scale_0_1 (SubVI).vi"("BLine D"=w776) -> ("Array"=w764:dbl[])  [unwired: 10 in]
                  n235 = Bundle By Name(cluster=w771, "Y"=w776) -> (w774:waveform(dbl))
                  n236 = Bundle By Name(cluster=w771, "Y"=w764) -> (w773:waveform(dbl))
                  n237 = Build Array (concatenate)(w753, w760, w764) -> (w763:dbl[][])
                }
                frame True {
                  (unwired) 0.0 ("T_Flow Start (s)")
                  w779 = 1.0 ("T_Flow Start (s)")
                  w780 = 0.0 ("T_Flow Start (s)")
                  # "LSP"
                  # "Type A or B"
                  n238 = call "Get 2-Rayleigh Parameters (SubVI).vi"("Flow Peak Amp."=w779, "T_Flow Start (s)"=w780, "T_Flow Peak (s)"=w787, "T_Ejection period (s)"=w782, "Pressure (mmHg)"=w785) -> ("Optimised Parameter"=w786:dbl[])  [unwired: 6 in]
                  n239 = call "Get 1-Rayleigh Parameters (SubVI).vi"("Flow Peak Amp."=w778, "T_Flow Start (s)"=w782, "T_Flow Peak (s)"=w783, "T_Ejection period (s)"=w784, "Pressure (mmHg)"=w785) -> ("Optimised Parameter"=w781:dbl[])  [unwired: 6 in]
                  n240 = Build Array (concatenate)(w786, w781) -> (w798:dbl[])
                  n241 = call "N_Rayleigh_Flow Model (SubVI).vi"("PSQ (ml/s)"=w779, "T_Flow Start"=w780, "Parameters (1XN)"=w786, "Pressure (mmHg)"=w785) -> ("Waveform Graph"=w788:dbl[][], "n-Rayleigh Model Flow"=w791:waveform(dbl))  [unwired: 4 in]
                  n242 = call "N_Rayleigh_Flow Model (SubVI).vi"("PSQ (ml/s)"=w778, "T_Flow Start"=w782, "Parameters (1XN)"=w781, "Pressure (mmHg)"=w785) -> ("Waveform Graph"=w790:dbl[][], "n-Rayleigh Model Flow"=w789:waveform(dbl))  [unwired: 4 in]
                  n243 = Unbundle By Name(w791) -> ("Y"=w803:dbl[], "dt"=w797:dbl)
                  n244 = Unbundle By Name(w789) -> ("Y"=w802:dbl[])
                  n245 = Compound Arithmetic op=ADD(w803, w802) -> (w795:dbl[])
                  n246 = call "Scale_0_1 (SubVI).vi"("BLine D"=w795) -> ("Array"=w794:dbl[])  [unwired: 10 in]
                  n247 = Multiply(x=w801, y=w794) -> (x*y=w800:dbl[])
                  n248 = call "Scale_0_1 (SubVI).vi"("BLine D"=w800) -> ("Array"=w793:dbl[])  [unwired: 10 in]
                  n249 = Bundle By Name("dt"=w797, "Y"=w800) -> (w796:waveform(dbl))  [unwired: 1 in]
                  n250 = Bundle By Name(cluster=w796, "Y"=w793) -> (w799:waveform(dbl))
                  n251 = Build Array (concatenate)(w788, w790, w793) -> (w792:dbl[][])
                }
              }
              "m-Ray" <- w720
              n252 = Unbundle By Name(w723) -> ("Y"=w747:dbl[])
              n253 = Unbundle By Name(w726) -> ("Y"=w748:dbl[])
              n254 = call "Peak_Base_Error_Check (SubVI).vi"("Model Flow"=w726, "T_Ejection Period (s)"=w728, "T_Flow Peak (s)"=w729) -> ("Error"=w749:dbl[])  [unwired: 5 in, 3 out]
              n255 = Merge Signals(w731, w730, w727) -> ()  [unwired: 1 out]
              n256 = Multiply(x=w749, y=1000.0 ("T_Flow Start (s)")) -> (x*y=w740:dbl[])
              n257 = call "Error Analysis (SubVI).vi"("Measured Wave"=w748, "Reference Wave"=w747) -> ("RMSE"=w738:dbl)  [unwired: 6 in, 3 out]
              n258 = Index Array(array=w740) -> (element #1=w746:dbl, element #2=w745:dbl)  [unwired: 2 in]
              n259 = Less Or Equal?(x=w745, y=2.0 ("T_Flow Start (s)")) -> (x <= y?=w741:bool)
              n260 = Less Or Equal?(x=w746, y=1.0 ("T_Flow Start (s)")) -> (x <= y?=w742:bool)
              n261 = And(x=w742, y=w741) -> ()  [unwired: 1 out]
              n262 = case shown="True" TRUE {
                tunnel: [T11."3-Rayleigh Model" ("Enum") T11."STOP" ("Enum")] -> w737
                frame False {
                }
                frame True {
                }
              }
              "True - Type A or B" <- w735
            }
            frame "3-Rayleigh Model" {
              (unwired) TRUE
              w808 = 0.0 ("T_Flow Start (s)")
              n263 = call "Get 3-Rayleigh Parameters(SubVI).vi"("Flow Peak Amp."=w807, "T_Flow Start (s)"=w808, "T_Flow Peak (s)"=w809, "T_Ejection period (s)"=w810, "Pressure (mmHg)"=w811) -> ("Optimised Parameter"=w806:dbl[])  [unwired: 6 in]
              n264 = call "N_Rayleigh_Flow Model (SubVI).vi"("PSQ (ml/s)"=w807, "T_Flow Start"=w808, "Parameters (1XN)"=w806, "Pressure (mmHg)"=w811) -> ("n-Rayleigh Model Flow"=w812:waveform(dbl))  [unwired: 4 in, 1 out]
              n265 = call "Peak_Base_Error_Check (SubVI).vi"("Model Flow"=w812, "T_Ejection Period (s)"=w810, "T_Flow Peak (s)"=w809) -> ("Error"=w827:dbl[])  [unwired: 5 in, 3 out]
              n266 = Unbundle By Name(w818) -> ("Y"=w825:dbl[])
              n267 = Unbundle By Name(w812) -> ("Y"=w826:dbl[])
              n268 = call "Error Analysis (SubVI).vi"("Measured Wave"=w826, "Reference Wave"=w825) -> ("RMSE"=w817:dbl)  [unwired: 6 in, 3 out]
              n269 = Multiply(x=w827, y=1000.0 ("T_Flow Start (s)")) -> (x*y=w816:dbl[])
              n270 = Index Array(array=w816) -> (element #1=w824:dbl, element #2=w823:dbl)  [unwired: 2 in]
              n271 = Less Or Equal?(x=w823, y=2.0 ("T_Flow Start (s)")) -> (x <= y?=w819:bool)
              n272 = Less Or Equal?(x=w824, y=1.0 ("T_Flow Start (s)")) -> (x <= y?=w820:bool)
              n273 = And(x=w820, y=w819) -> (x .and. y?=w813:bool)
              n274 = case shown="True" w813 {
                tunnel: [T11."4-Rayeligh Model" ("Enum") T11."STOP" ("Enum")] -> w814
                frame False {
                }
                frame True {
                }
              }
            }
            frame "4-Rayeligh Model" {
              w833 = 0.0 ("T_Flow Start (s)")
              n275 = call "Get 4-Rayleigh Parameters(SubVI).vi"("Flow Peak Amp."=w832, "T_Flow Start (s)"=w833, "T_Flow Peak (s)"=w834, "T_Ejection period (s)"=w835, "Pressure (mmHg)"=w836) -> ("Optimised Parameter"=w831:dbl[])  [unwired: 6 in]
              n276 = call "N_Rayleigh_Flow Model (SubVI).vi"("PSQ (ml/s)"=w832, "T_Flow Start"=w833, "Parameters (1XN)"=w831, "Pressure (mmHg)"=w836) -> ("n-Rayleigh Model Flow"=w837:waveform(dbl))  [unwired: 4 in, 1 out]
              n277 = call "Peak_Base_Error_Check (SubVI).vi"("Model Flow"=w837, "T_Ejection Period (s)"=w835, "T_Flow Peak (s)"=w834) -> ("Error"=w852:dbl[])  [unwired: 5 in, 3 out]
              n278 = Unbundle By Name(w843) -> ("Y"=w850:dbl[])
              n279 = Unbundle By Name(w837) -> ("Y"=w851:dbl[])
              n280 = call "Error Analysis (SubVI).vi"("Measured Wave"=w851, "Reference Wave"=w850) -> ("RMSE"=w842:dbl)  [unwired: 6 in, 3 out]
              n281 = Multiply(x=w852, y=1000.0 ("T_Flow Start (s)")) -> (x*y=w841:dbl[])
              n282 = Index Array(array=w841) -> (element #1=w849:dbl, element #2=w848:dbl)  [unwired: 2 in]
              n283 = Less Or Equal?(x=w848, y=2.0 ("T_Flow Start (s)")) -> (x <= y?=w844:bool)
              n284 = Less Or Equal?(x=w849, y=1.0 ("T_Flow Start (s)")) -> (x <= y?=w845:bool)
              n285 = And(x=w845, y=w844) -> (x .and. y?=w838:bool)
              n286 = case shown="True" w838 {
                tunnel: [T11."5-Rayleigh Model" ("Enum") T11."STOP" ("Enum")] -> w839
                frame False {
                }
                frame True {
                }
              }
            }
            frame "5-Rayleigh Model" {
              w858 = 0.0 ("T_Flow Start (s)")
              n287 = call "Get 5-Rayleigh Parameters(SubVI).vi"("Flow Peak Amp."=w856, "T_Flow Start (s)"=w858, "T_Flow Peak (s)"=w859, "T_Ejection period (s)"=w860, "Pressure (mmHg)"=w861) -> ("Optimised Parameter"=w857:dbl[])  [unwired: 6 in]
              n288 = call "N_Rayleigh_Flow Model (SubVI).vi"("PSQ (ml/s)"=w856, "T_Flow Start"=w858, "Parameters (1XN)"=w857, "Pressure (mmHg)"=w861) -> ("n-Rayleigh Model Flow"=w862:waveform(dbl))  [unwired: 4 in, 1 out]
              n289 = call "Peak_Base_Error_Check (SubVI).vi"("Model Flow"=w862, "T_Ejection Period (s)"=w860, "T_Flow Peak (s)"=w859) -> ("Error"=w875:dbl[])  [unwired: 5 in, 3 out]
              n290 = Unbundle By Name(w866) -> ("Y"=w873:dbl[])
              n291 = Unbundle By Name(w862) -> ("Y"=w874:dbl[])
              n292 = call "Error Analysis (SubVI).vi"("Measured Wave"=w874, "Reference Wave"=w873) -> ("RMSE"=w865:dbl)  [unwired: 6 in, 3 out]
              n293 = Multiply(x=w875, y=1000.0 ("T_Flow Start (s)")) -> (x*y=w864:dbl[])
              n294 = Index Array(array=w864) -> (element #1=w872:dbl, element #2=w871:dbl)  [unwired: 2 in]
              n295 = Less Or Equal?(x=w871, y=2.0 ("T_Flow Start (s)")) -> (x <= y?=w867:bool)
              n296 = Less Or Equal?(x=w872, y=1.0 ("T_Flow Start (s)")) -> (x <= y?=w868:bool)
              n297 = And(x=w868, y=w867) -> ()  [unwired: 1 out]
            }
            frame "STOP" {
            }
          }
        }
        "Model Optimised Parameter" <- w617
        "Model Error (ms)" <- w608
        "RMSE Ray Model" <- w618
        "#Rayeligh" <- w619
        n298 = call "Tri. Flow Model (SubVI).vi"("Offset"=0.0, "T_Flow Start (s)"=0.0, "T_Ejection Period (s)"=w656, "Pressure (mmHg)"=w659, "T_Flow Peak (s)"=w658, "Flow Amp."=w657) -> ("Triangular  Model Flow"=w622:waveform(dbl))  [unwired: 5 in]
        n299 = Unbundle By Name(w629) -> ("Y"=w640:dbl[], "dt"=w653:dbl)
        n300 = Unbundle By Name(w627) -> ("Y"=w637:dbl[], "dt"=w652:dbl)
        n301 = Unbundle By Name(w622) -> ("Y"=w638:dbl[], "dt"=w651:dbl)
        n302 = Merge Signals(w634, w633, w629, w627, w622) -> (→"Flow Rate Model":dynamicdata)
        n303 = Array Subset(array=w640, length=w639) -> (w636:dbl[])  [unwired: 1 in]
        n304 = Array Subset(array=w637, length=w639) -> (w635:dbl[])  [unwired: 1 in]
        n305 = Array Subset(array=w638, length=w639) -> ()  [unwired: 1 in, 1 out]
        n306 = Unbundle By Name(w630) -> ("Flow Velocity (m/s)"=w628:waveform(dbl), "Area (mm^2)"=w631:waveform(dbl))
        n307 = call <vilib>:"Correlation Coefficient.vi"("Y"=w635, "X"=w636) -> ("correlation coefficient r"=w612:dbl)  [unwired: 8 in, 1 out]
        "correlation coefficient r" <- w612
        n308 = call <vilib>:"Amplitude and Phase Spectrum.vi"("dt"=w653, "Signal (V)"=w640) -> ("df"=w649:dbl, "Amp Spectrum Mag (Vrms)"=w650:dbl[])  [unwired: 1 in, 1 out]
        n309 = call <vilib>:"Amplitude and Phase Spectrum.vi"("dt"=w652, "Signal (V)"=w637) -> ("df"=w645:dbl, "Amp Spectrum Mag (Vrms)"=w646:dbl[])  [unwired: 1 in, 1 out]
        n310 = call <vilib>:"Amplitude and Phase Spectrum.vi"("dt"=w651, "Signal (V)"=w638) -> ("df"=w643:dbl, "Amp Spectrum Mag (Vrms)"=w644:dbl[])  [unwired: 1 in, 1 out]
        n311 = Bundle By Name("Y"=w650, "dt"=w649) -> (w647:waveform(dbl))  [unwired: 1 in]
        n312 = Bundle By Name("Y"=w646, "dt"=w645) -> (w642:waveform(dbl))  [unwired: 1 in]
        n313 = Bundle By Name("Y"=w644, "dt"=w643) -> (w641:waveform(dbl))  [unwired: 1 in]
        n314 = Build Array (concatenate)(w612, w619, w618, w608, w617) -> (w616:dbl[])
        n315 = Merge Signals(w647, w642, w641) -> (→"Magnitude Spectrum Flow":dynamicdata)
        n316 = call "Min_Max_Amp (SubVI).vi"("waveform"=w631) -> ("MN"=w632:dbl)  [unwired: 8 in, 2 out]
        n317 = Divide(x=w632, y=w623) -> (x/y=w620:dbl)
        n318 = Divide(x=w627, y=w623) -> (x/y=w626:waveform(dbl))
        n319 = Divide(x=w622, y=w623) -> (x/y=w624:waveform(dbl))
        n320 = Divide(x=w626, y=w620) -> (x/y=w625:waveform(dbl))
        n321 = Divide(x=w624, y=w620) -> (x/y=w621:waveform(dbl))
        "mean" <- w600
        "SDW ZC 2" <- w598
        "mean 2" <- w599
      }
      frame #4 {
        n322 = Unbundle By Name(w983) -> ("Y"=w989:dbl[])
        n323 = Unbundle By Name(w948) -> ("Y"=w988:dbl[])
        n324 = Unbundle By Name(w983) -> ("Y"=w987:dbl[])
        n325 = Unbundle By Name(w947) -> ("Y"=w986:dbl[])
        n326 = Unbundle By Name(w983) -> ("Y"=w985:dbl[])
        n327 = Unbundle By Name(w946) -> ("Y"=w984:dbl[])
        n328 = call "PWV_dPdU(SubVI).vi"("Flow Velocity (m/s)"=w988, "Pressure (mmHg)"=w989) -> ("PWV (m/s) (dPdU)"=w916:dbl)  [unwired: 9 in]
        n329 = call "PWV_dPdU(SubVI).vi"("Flow Velocity (m/s)"=w986, "Pressure (mmHg)"=w987) -> ("PWV (m/s) (dPdU)"=w915:dbl)  [unwired: 9 in]
        n330 = call "PWV_dPdU(SubVI).vi"("Flow Velocity (m/s)"=w984, "Pressure (mmHg)"=w985) -> ("PWV (m/s) (dPdU)"=w914:dbl)  [unwired: 9 in]
        n331 = call "Input Impedence_Freq Domian(SubVI).vi"("Settings"="Settings 2", "Flow Rate (ml/s)"=w899, "Pressure (mmHg)"=w983) -> ("Zo (at 0 Hz) (mmHg/ml/s)"=w924:dbl, "Zc (mmHg/ml/s)"=w925:dbl)  [unwired: 5 in, 2 out]
        "Zc FD (mmHg/ml/s) - Reference" <- w925
        "PVR (mmHg/ml/s) - Reference" <- w924
        n332 = call "Input Impedence_Freq Domian(SubVI).vi"("Settings"="Settings 2", "Flow Rate (ml/s)"=w898, "Pressure (mmHg)"=w983) -> ("Zo (at 0 Hz) (mmHg/ml/s)"=w922:dbl, "Zc (mmHg/ml/s)"=w923:dbl, "Zo - Magnitude Spectrum"=→"Input Impedence - Magnitude Spectrum  2":waveform(dbl))  [unwired: 5 in, 1 out]
        "Zc FD (mmHg/ml/s) - Rayleigh" <- w923
        "PVR (mmHg/ml/s) - Rayleigh" <- w922
        n333 = call "Input Impedence_Freq Domian(SubVI).vi"("Settings"="Settings 2", "Flow Rate (ml/s)"=w982, "Pressure (mmHg)"=w983) -> ("Zo (at 0 Hz) (mmHg/ml/s)"=w920:dbl, "Zc (mmHg/ml/s)"=w921:dbl)  [unwired: 5 in, 2 out]
        "PVR (mmHg/ml/s) - Triangular" <- w920
        "Zc FD (mmHg/ml/s) - Triangular" <- w921
        n334 = call "Input Impedence_Time Domain(SubVI).vi"("Ad (m^2)"=w949, "PWV (m/s)"=w916) -> ("Zc (mmHg/ml/s)"=w919:dbl)  [unwired: 9 in]
        "Zc TD (mmHg/ml/s) - Reference" <- w919
        n335 = call "Input Impedence_Time Domain(SubVI).vi"("Ad (m^2)"=w949, "PWV (m/s)"=w915) -> ("Zc (mmHg/ml/s)"=w918:dbl)  [unwired: 9 in]
        "Zc TD (mmHg/ml/s) - Rayleigh" <- w918
        n336 = call "Input Impedence_Time Domain(SubVI).vi"("Ad (m^2)"=w949, "PWV (m/s)"=w914) -> ("Zc (mmHg/ml/s)"=w917:dbl)  [unwired: 9 in]
        "Zc TD (mmHg/ml/s) - Triangular" <- w917
        n337 = Build Array(w925, w924, w923, w922, w921, w920, w919, w918, w917, w916, w915, w914) -> (w913:dbl[])
        n338 = call "Classical WSA (SubVI).vi"("Zc (mmHg/ml/s)"=w925, "Flow Rate (ml/s)"=w899, "Pressure (mmHg)"=w983) -> ("WSA Waveforms"=w981:T14)  [unwired: 8 in]
        n339 = call "Classical WSA (SubVI).vi"("Zc (mmHg/ml/s)"=w919, "Flow Rate (ml/s)"=w899, "Pressure (mmHg)"=w983) -> ("WSA Waveforms"=w980:T14)  [unwired: 8 in]
        n340 = call "Classical WSA (SubVI).vi"("Zc (mmHg/ml/s)"=w923, "Flow Rate (ml/s)"=w898, "Pressure (mmHg)"=w983) -> ("WSA Waveforms"=w976:T14)  [unwired: 8 in]
        n341 = call "Classical WSA (SubVI).vi"("Zc (mmHg/ml/s)"=w918, "Flow Rate (ml/s)"=w898, "Pressure (mmHg)"=w983) -> ("WSA Waveforms"=w977:T14)  [unwired: 8 in]
        n342 = call "Classical WSA (SubVI).vi"("Zc (mmHg/ml/s)"=w921, "Flow Rate (ml/s)"=w982, "Pressure (mmHg)"=w983) -> ("WSA Waveforms"=w978:T14)  [unwired: 8 in]
        n343 = call "Classical WSA (SubVI).vi"("Zc (mmHg/ml/s)"=w917, "Flow Rate (ml/s)"=w982, "Pressure (mmHg)"=w983) -> ("WSA Waveforms"=w979:T14)  [unwired: 8 in]
        n344 = Unbundle By Name(w899) -> ("Y"=w897:dbl[])
        n345 = Unbundle By Name(w898) -> ("Y"=w896:dbl[])
        n346 = Unbundle By Name(w981) -> ("P FWD"=w902:waveform(dbl), "P BWD"=w959:waveform(dbl))
        n347 = Unbundle By Name(w978) -> ("P FWD"=w953:waveform(dbl), "P BWD"=w952:waveform(dbl))
        n348 = Unbundle By Name(w980) -> ("P FWD"=w958:waveform(dbl), "P BWD"=w957:waveform(dbl))
        n349 = Unbundle By Name(w979) -> ("P FWD"=w951:waveform(dbl), "P BWD"=w950:waveform(dbl))
        n350 = Unbundle By Name(w976) -> ("P FWD"=w901:waveform(dbl), "P BWD"=w956:waveform(dbl))
        n351 = Unbundle By Name(w977) -> ("P FWD"=w955:waveform(dbl), "P BWD"=w954:waveform(dbl))
        n352 = call "Error Analysis (SubVI).vi"("Measured Wave"=w896, "Reference Wave"=w897) -> ("RMSE"=w895:dbl)  [unwired: 6 in, 3 out]
        n353 = call "RTT_XCorr_Method (SubVI).vi"("P BWD"=w959, "P FWD"=w902) -> ("RTT (ms)"=w945:dbl)  [unwired: 9 in]
        "Ref. RWTT XCorr (FD)(ms)" <- w945
        n354 = call "RTT_ZC_Method (SubVI).vi"("P BWD"=w959, "P FWD"=w902) -> ("RTT (ms)"=w944:dbl)  [unwired: 9 in]
        "Ref. RWTT ZC (FD)(ms)" <- w944
        n355 = call "RTT_XCorr_Method (SubVI).vi"("P BWD"=w957, "P FWD"=w958) -> ("RTT (ms)"=w943:dbl)  [unwired: 9 in]
        "Ref. RWTT XCorr (TD)(ms)" <- w943
        n356 = call "RTT_ZC_Method (SubVI).vi"("P BWD"=w957, "P FWD"=w958) -> ("RTT (ms)"=w942:dbl)  [unwired: 9 in]
        "Ref. RWTT ZC (TD)(ms)" <- w942
        n357 = call "RTT_XCorr_Method (SubVI).vi"("P BWD"=w956, "P FWD"=w901) -> ("RTT (ms)"=w941:dbl)  [unwired: 9 in]
        "m-Ray RWTT XCorr (FD)(ms)" <- w941
        n358 = call "RTT_ZC_Method (SubVI).vi"("P BWD"=w956, "P FWD"=w901) -> ("RTT (ms)"=w940:dbl)  [unwired: 9 in]
        "m-Ray RWTT ZC (FD)(ms)" <- w940
        n359 = call "RTT_XCorr_Method (SubVI).vi"("P BWD"=w954, "P FWD"=w955) -> ("RTT (ms)"=w939:dbl)  [unwired: 9 in]
        "m-Ray RWTT XCorr (TD)(ms)" <- w939
        n360 = call "RTT_ZC_Method (SubVI).vi"("P BWD"=w954, "P FWD"=w955) -> ("RTT (ms)"=w938:dbl)  [unwired: 9 in]
        "m-Ray RWTT ZC (TD)(ms)" <- w938
        n361 = call "RTT_XCorr_Method (SubVI).vi"("P BWD"=w952, "P FWD"=w953) -> ("RTT (ms)"=w937:dbl)  [unwired: 9 in]
        "Tri.  RWTT XCorr (FD)(ms)" <- w937
        n362 = call "RTT_ZC_Method (SubVI).vi"("P BWD"=w952, "P FWD"=w953) -> ("RTT (ms)"=w936:dbl)  [unwired: 9 in]
        "Tri.  RWTT ZC (FD)(ms)" <- w936
        n363 = call "RTT_XCorr_Method (SubVI).vi"("P BWD"=w950, "P FWD"=w951) -> ("RTT (ms)"=w935:dbl)  [unwired: 9 in]
        "Tri.  RWTT XCorr (TD)(ms)" <- w935
        n364 = call "RTT_ZC_Method (SubVI).vi"("P BWD"=w950, "P FWD"=w951) -> ("RTT (ms)"=w934:dbl)  [unwired: 9 in]
        "Tri.  RWTT  ZC (TD)(ms)" <- w934
        n365 = call "Min_Max_Amp (SubVI).vi"("waveform"=w901) -> ()  [unwired: 8 in, 3 out]
        n366 = call "Min_Max_Amp (SubVI).vi"("waveform"=w902) -> ()  [unwired: 8 in, 3 out]
        n367 = Merge Signals(w958, w955, w951) -> (→"Forward Pressure Wave (Time Domain Analysis)":dynamicdata)
        n368 = Merge Signals(w957, w954, w950) -> (→"Backward Pressure Wave (Time Domain Analysis)":dynamicdata)
        n369 = Merge Signals(w959, w956, w952) -> (→"Backward Pressure Wave (Freq. Domain Analysis)":dynamicdata)
        n370 = Merge Signals(w902, w901, w953) -> (→"Forward Pressure Wave (Freq. Domain Analysis)":dynamicdata)
        n371 = Build Array(w945, w944, w943, w942, w941, w940, w939, w938, w937, w936, w935, w934) -> (w926:dbl[])
        n372 = Unbundle By Name(w959) -> ("Y"=w967:dbl[])
        n373 = Unbundle By Name(w958) -> ("Y"=w964:dbl[])
        n374 = Unbundle By Name(w957) -> ("Y"=w961:dbl[])
        n375 = Unbundle By Name(w901) -> ("Y"=w970:dbl[])
        n376 = Unbundle By Name(w956) -> ("Y"=w968:dbl[])
        n377 = Unbundle By Name(w955) -> ("Y"=w965:dbl[])
        n378 = Unbundle By Name(w954) -> ("Y"=w962:dbl[])
        n379 = Unbundle By Name(w953) -> ("Y"=w969:dbl[])
        n380 = Unbundle By Name(w952) -> ("Y"=w966:dbl[])
        n381 = Unbundle By Name(w951) -> ("Y"=w963:dbl[])
        n382 = Unbundle By Name(w950) -> ("Y"=w960:dbl[])
        n383 = Unbundle By Name(w902) -> ("Y"=w971:dbl[])
        n384 = call "Error Analysis (SubVI).vi"("Measured Wave"=w970, "Reference Wave"=w971) -> ("RMSE"=w893:dbl)  [unwired: 6 in, 3 out]
        "RMSE (Fwd Rayleigh FD)" <- w893
        n385 = call "Error Analysis (SubVI).vi"("Measured Wave"=w969, "Reference Wave"=w971) -> ("RMSE"=w933:dbl)  [unwired: 6 in, 3 out]
        "RMSE (Fwd Triangular FD)" <- w933
        n386 = call "Error Analysis (SubVI).vi"("Measured Wave"=w968, "Reference Wave"=w967) -> ("RMSE"=w892:dbl)  [unwired: 6 in, 3 out]
        "RMSE (Bwd Rayleigh FD)" <- w892
        n387 = call "Error Analysis (SubVI).vi"("Measured Wave"=w966, "Reference Wave"=w967) -> ("RMSE"=w932:dbl)  [unwired: 6 in, 3 out]
        "RMSE (Bwd Triangular FD)" <- w932
        n388 = call "Error Analysis (SubVI).vi"("Measured Wave"=w965, "Reference Wave"=w964) -> ("RMSE"=w931:dbl)  [unwired: 6 in, 3 out]
        "RMSE (Fwd Rayleigh TD)" <- w931
        n389 = call "Error Analysis (SubVI).vi"("Measured Wave"=w963, "Reference Wave"=w964) -> ("RMSE"=w930:dbl)  [unwired: 6 in, 3 out]
        "RMSE (Fwd Triangular TD)" <- w930
        n390 = call "Error Analysis (SubVI).vi"("Measured Wave"=w962, "Reference Wave"=w961) -> ("RMSE"=w929:dbl)  [unwired: 6 in, 3 out]
        "RMSE (Bwd Rayleigh TD)" <- w929
        n391 = call "Error Analysis (SubVI).vi"("Measured Wave"=w960, "Reference Wave"=w961) -> ("RMSE"=w928:dbl)  [unwired: 6 in, 3 out]
        "RMSE (Bwd Triangular TD)" <- w928
        n392 = call "Get RM_RI (SubVI).vi"("Bwd"=w967, "Fwd"=w971) -> ("Reflection Markers"=w908:T15)  [unwired: 9 in]
        "Reference (FD)" <- w908
        n393 = call "Get RM_RI (SubVI).vi"("Bwd"=w961, "Fwd"=w964) -> ("Reflection Markers"=w907:T15)  [unwired: 9 in]
        "Reference (TD)" <- w907
        n394 = call "Get RM_RI (SubVI).vi"("Bwd"=w968, "Fwd"=w970) -> ("Reflection Markers"=w906:T15)  [unwired: 9 in]
        "Rayleigh (FD)" <- w906
        n395 = call "Get RM_RI (SubVI).vi"("Bwd"=w962, "Fwd"=w965) -> ("Reflection Markers"=w905:T15)  [unwired: 9 in]
        "Rayleigh (TD)" <- w905
        n396 = call "Get RM_RI (SubVI).vi"("Bwd"=w966, "Fwd"=w969) -> ("Reflection Markers"=w904:T15)  [unwired: 9 in]
        "Triangular (FD)" <- w904
        n397 = call "Get RM_RI (SubVI).vi"("Bwd"=w960, "Fwd"=w963) -> ("Reflection Markers"=w903:T15)  [unwired: 9 in]
        "Triangular (TD)" <- w903
        n398 = Build Array(w893, w933, w892, w932, w931, w930, w929, w928) -> (w927:dbl[])
      }
    }
    n399 = Unbundle(w207) -> ("del Pf (mmHg)"=w227:dbl, "del Pb (mmHg)"=w225:dbl, "RM"=w124:dbl, "RI (%)"=w226:dbl)
    n400 = Unbundle(w206) -> ("del Pf (mmHg)"=w224:dbl, "del Pb (mmHg)"=w223:dbl, "RM"=w222:dbl, "RI (%)"=w221:dbl)
    n401 = Unbundle(w205) -> ("del Pf (mmHg)"=w220:dbl, "del Pb (mmHg)"=w219:dbl, "RM"=w123:dbl, "RI (%)"=w218:dbl)
    n402 = Unbundle(w204) -> ("del Pf (mmHg)"=w217:dbl, "del Pb (mmHg)"=w216:dbl, "RM"=w215:dbl, "RI (%)"=w126:dbl)
    n403 = Unbundle(w203) -> ("del Pf (mmHg)"=w214:dbl, "del Pb (mmHg)"=w213:dbl, "RM"=w212:dbl, "RI (%)"=w211:dbl)
    n404 = Unbundle(w202) -> ("del Pf (mmHg)"=w210:dbl, "del Pb (mmHg)"=w209:dbl, "RM"=w208:dbl, "RI (%)"=w200:dbl)
    n405 = Index Array(array=w201) -> (element #1=w198:dbl, element #2=w197:dbl, element #3=w196:dbl, element #4=w195:dbl, element #5=w194:dbl, element #6=w193:dbl, element #7=w192:dbl, element #8=w199:dbl)  [unwired: 8 in]
    n406 = Index Array(array=w183) -> (element #1=w190:dbl, element #2=w189:dbl, element #3=w188:dbl, element #4=w187:dbl, element #5=w186:dbl, element #6=w185:dbl, element #7=w184:dbl, element #8=w191:dbl, element #9=w179:dbl, element #10=w180:dbl, element #11=w181:dbl, element #12=w182:dbl)  [unwired: 12 in]
    n407 = Unbundle(w229) -> ("SF"=w243:dbl, "ER"=w242:dbl, "IP"=w241:dbl, "DN"=w240:dbl, "SDW ZC 1"=w239:dbl, "MX"=w238:dbl, "FDW ZC"=w237:dbl, "FoDW ZC"=w236:dbl)  [unwired: 1 out]
    n408 = Unbundle(w228) -> ("Type (4th D ZC)"=w235:enum16{"Type A", "Type B", "Type C"}, "AIx (%) (4th D ZC)"=w103:dbl, "AP (mmHg)  (4th DZC)"=w234:dbl)
    n409 = Index Array(array=w168) -> (element #1=w177:dbl, element #2=w122:dbl, element #3=w176:dbl, element #4=w175:dbl, element #5=w174:dbl, element #6=w121:dbl, element #7=w173:dbl, element #8=w178:dbl, element #9=w169:dbl, element #10=w170:dbl, element #11=w171:dbl, element #12=w172:dbl)  [unwired: 12 in]
    n410 = Index Array(array=w152) -> (element #1=w151:dbl, element #2=w142:dbl, element #3=w143:dbl, element #4=w144:dbl, element #5=w145:dbl, element #6=w146:dbl, element #7=w147:dbl, element #8=w148:dbl, element #9=w149:dbl, element #10=w150:dbl)  [unwired: 10 in]
    n411 = Index Array(array=w160) -> (element #1=w104:dbl, element #2=w166:dbl, element #3=w165:dbl, element #4=w164:dbl, element #5=w163:dbl, element #6=w162:dbl, element #7=w161:dbl, element #8=w167:dbl)  [unwired: 8 in]
    n412 = Index Array(array=w153) -> (element #1=w154:dbl, element #2=w159:dbl, element #3=w158:dbl, element #4=w157:dbl, element #5=w156:dbl, element #6=w155:dbl)  [unwired: 6 in]
    n413 = Unbundle(w95) -> ("MX (s)"=w94:dbl, "SD ZC 1 (s)"=w93:dbl, "FoDW ZC (s)"=w92:dbl, "IP (s)"=w91:dbl, "DN (s)"=w90:dbl)  [unwired: 1 out]
    n414 = Merge Signals(w94, w93, w92, w91, w90) -> (w233:dynamicdata)
    n415 = Merge Signals(w243, w242, w241, w240, w239, w238, w237, w236) -> (w230:dynamicdata)
    n416 = Merge Signals(w235, w103, w234) -> (w137:dynamicdata)
    n417 = Merge Signals(w227, w225, w124, w226) -> (w136:dynamicdata)
    n418 = Merge Signals(w224, w223, w222, w221) -> (w135:dynamicdata)
    n419 = Merge Signals(w220, w219, w123, w218) -> (w134:dynamicdata)
    n420 = Merge Signals(w217, w216, w215, w126) -> (w133:dynamicdata)
    n421 = Merge Signals(w214, w213, w212, w211) -> (w132:dynamicdata)
    n422 = Merge Signals(w210, w209, w208, w200) -> (w131:dynamicdata)
    n423 = Merge Signals(w198, w197, w196, w195, w194, w193, w192, w199) -> (w130:dynamicdata)
    n424 = Merge Signals(w190, w189, w188, w187, w186, w185, w184, w191, w179, w180, w181, w182) -> (w129:dynamicdata)
    n425 = Merge Signals(w177, w122, w176, w175, w174, w121, w173, w178, w169, w170, w171, w172) -> (w128:dynamicdata)
    n426 = Merge Signals(w151, w142, w143, w144, w145, w146, w147, w148, w149, w150) -> (w127:dynamicdata)
    n427 = Merge Signals(w154, w159, w158, w157, w156, w155) -> (w140:dynamicdata)
    n428 = Merge Signals(w104, w166, w165, w164, w163, w162, w161, w167) -> (w141:dynamicdata)
    n429 = Multiply(x=w233, y=1000.0 ("Max. Freq. for Zc")) -> (x*y=w139:dynamicdata)
    n430 = Multiply(x=w230, y=1000.0 ("Max. Freq. for Zc")) -> (x*y=w138:dynamicdata)
    n431 = Merge Signals(w268, w141, w140, w139, w138, w137, w136, w135, w134, w133, w132, w131, w130, w129, w128, w127) -> (w269:dynamicdata)
    n432 = call "Write To Measurement File"("Signals"=w269, "Reset"="Save Data", "Enable"="Save Data", "Filename"="File to Save Data") -> ("Saving Data"=→"Saving Data":bool)  [unwired: 13 in, 2 out]
    n433 = Tick Count (ms)() -> (millisecond timer value=w278:u32)
    n434 = Index Array(array=w112) -> (element #1=w111:dbl, element #2=w110:dbl)  [unwired: 2 in]
  }
  "Array" <- w1
  n435 = call-poly <vilib>:"Mean.vi"("X"=w15) -> ("mean"=→"mean RMSE PF":dbl)  [unwired: 1 out]
  n436 = call-poly <vilib>:"Mean.vi"("X"=w18) -> ("mean"=→"mean RMSE PB":dbl)  [unwired: 1 out]
  n437 = Subtract(x=w31, y=w30) -> (x-y=w26:dbl[])
  n438 = Add(x=w31, y=w30) -> (x+y=w29:dbl[])
  n439 = call-poly <vilib>:"Mean.vi"("X"=w24) -> ("mean"=→"mean RMSE for Q":dbl)  [unwired: 1 out]
  n440 = call-poly <vilib>:"Mean.vi"("X"=w22) -> ("mean"=→"mean Peak err":dbl)  [unwired: 1 out]
  n441 = call-poly <vilib>:"Mean.vi"("X"=w21) -> ("mean"=→"mean base err":dbl)  [unwired: 1 out]
  n442 = call <vilib>:"Correlation Coefficient.vi"("Y"=w34, "X"=w35) -> ("correlation coefficient r"=→"correlation coefficient r 3":dbl)  [unwired: 8 in, 1 out]
  n443 = Divide(x=w29, y=2.0 ("Max. Freq. for Zc")) -> (x/y=w27:dbl[])
  n444 = call <vilib>:"Linear Fit.vi"("Y"=w7, "X"=w14) -> ("Best Linear Fit"=w13:dbl[], "slope"=→"slope":dbl, "intercept"=→"intercept":dbl)  [unwired: 9 in, 2 out]
  n445 = call <vilib>:"Correlation Coefficient.vi"("Y"=w30, "X"=w31) -> ("correlation coefficient r"=→"correlation coefficient r 2":dbl)  [unwired: 8 in, 1 out]
  n446 = call <vilib>:"Linear Fit.vi"("Y"=w7, "X"=w6) -> ("Best Linear Fit"=w5:dbl[])  [unwired: 9 in, 4 out]
  n447 = Bundle(w35, w34) -> (→"XY Graph 2":cluster{dbl[], dbl[]})  [unwired: 1 in]
  n448 = Bundle(w31, w30) -> (→"XY Graph":cluster{dbl[], dbl[]})  [unwired: 1 in]
  n449 = Bundle(w14, w7) -> (w12:cluster{dbl[], dbl[]})  [unwired: 1 in]
  n450 = Bundle(w14, "Best Linear Fit"=w13) -> (w11:cluster{dbl[], "Best Linear Fit":dbl[]})  [unwired: 1 in]
  n451 = Bundle(w6, w7) -> (w4:cluster{dbl[], dbl[]})  [unwired: 1 in]
  n452 = Bundle(w6, "Best Linear Fit"=w5) -> (w3:cluster{dbl[], "Best Linear Fit":dbl[]})  [unwired: 1 in]
  n453 = Bundle(w27, w26) -> (→"XY Graph 3":cluster{dbl[], dbl[]})  [unwired: 1 in]
  n454 = Build Array(w12, w11) -> (→"A2/A1 vs Age":cluster{dbl[], "Best Linear Fit":dbl[]}[])
  n455 = Build Array(w4, w3) -> (→"A2/A1 vs. AIx":cluster{dbl[], "Best Linear Fit":dbl[]}[])
